vi "MultiPAS-IV_noCRD.vi"() -> ()   [LabVIEW 2011]
uses:
  <vilib>/Analysis/4window.llb/windowTd.ctl
  sub/QMH/QMH Add Message to Queue (Single Element).vi
  sub/QMH/QMH Add Message to Queue (Array).vi
  <vilib>/measure/maspectr.llb/FFT Spectrum (Mag-Phase) for 1 Chan.vi
  <vilib>/Instr/_visa.llb/VISA Configure Serial Port (Instr).vi
  <vilib>/measure/NI_MAPro.lvlib
  <vilib>/Analysis/NI_AALPro.lvlib
panel:
  in  "785 Power (mW)":dbl(slide)=100.0 min=0.0 max=100.0 step=1.0 scale=0.0..100.0
  in  "785 Emission":bool
  out "PAS Save":bool caption="Overtemp"
  in  "Data 2":i32[][](array[numeric])=[[-16374, -7248, 2543, 12030, 20279, 26487, 30037, 30583, 28073, 22744, 15131, 5976, -3818, -13288, -21504, -27663, -31155, -31636, -29064, -23686, -16036, -6862, 2936, 12388, 20571, 26684, 30122, 30546, 27911, 22483, 14793, 5595, -4207, -13644, -21795, -27855, -31232, -31591, -28898, -23423, -15695, -6476, 3323, 12743, 20858, 26873, 30194, 30492, 27744, 22213, 14447, 5207, -4597, -14002, -22082, -28044, -31304, -31540, -28731, -23149, -15348, -6093, 3713, 13101, 21145, 27063, 30265, 30442, 27576, 21943, 14103, 4822, -4984, -14354, -22365, -28230, -31373, -31485, -28556, -22876, -14998, -5702, 4104, 13452, 21428, 27245, 30335, 30388, 27400, 21669, 13754, 4435, -5375, -14705, -22643, -28407, -31436, -31426, -28378, -22598, -14648, -5314, 4497, 13803, 21706, 27423, 30394, 30325, 27221, 21390, 13402, 4045, -5763, -15056, -22921, -28586, -31496, -31361, -28198, -22319, -14297, -4924, 4879, 14151, 21982, 27597, 30451, 30257, 27038, 21107, 13050, 3658, -6149, -15402, -23193, -28754, -31546, -31290, -28010, -22033, -13944, -4536, 5266, 14498, 22252, 27767, 30500, 30184, 26849, 20821, 12696, 3267, -6535, -15748, -23462, -28924, -31596, -31216, -27821, -21748, -13587, -4147, 5653, 14838, 22519, 27930, 30549, 30110, 26658, 20535, 12337, 2878, -6919, -16089, -23727, -29087, -31641, -31137, -27627, -21457, -13229, -3753, 6038, 15181, 22786, 28093, 30591, 30031, 26461, 20243, 11979, 2485, -7303, -16428, -23991, -29244, -31678, -31053, -27426, -21159, -12867, -3360, 6424, 15524, 23043, 28252, 30633, 29946, 26262, 19946, 11617, 2096, -7686, -16764, -24246, -29398, -31712, -30964, -27224, -20862, -12503, -2971, 6803, 15859, 23301, 28401, 30661, 29852, 26058, 19648, 11254, 1703, -8069, -17099, -24500, -29547, -31741, -30870, -27018, -20562, -12138, -2575, 7188, 16192, 23556, 28549, 30689, 29756, 25848, 19348, 10891, 1312, -8448, -17430, -24753, -29691, -31765, -30773, -26806, -20259, -11775, -2186, 7566, 16521, 23801, 28690, 30709, 29656, 25634, 19038, 10523, 919, -8831, -17762, -24997, -29833, -31788, -30672, -26593, -19955, -11409, -1792, 7944, 16850, 24047, 28830, 30724, 29548, 25416, 18729, 10152, 523, -9212, -18092, -25245, -29969, -31805, -30566, -26375, -19647, -11041, -1403, 8319, 17173, 24287, 28963, 30734, 29436, 25192, 18418, 9781, 130, -9587, -18413, -25481, -30101, -31814, -30449, -26150, -19332, -10666, -1007, 8697, 17497, 24524, 29090, 30745, 29325, 24968, 18105, 9408, -263, -9962, -18735, -25718, -30228, -31820, -30334, -25921, -19016, -10296, -618, 9072, 17814, 24756, 29213, 30746, 29202, 24738, 17787, 9036, -657, -10338, -19058, -25951, -30350, -31818, -30214, -25690, -18699, -9922, -224, 9442, 18128, 24984, 29330, 30738, 29078, 24502, 17466, 8658, -1050, -10710, -19371, -26178, -30467, -31814, -30088, -25458, -18382, -9550, 167, 9812, 18440, 25206, 29443, 30732, 28947, 24264, 17143, 8281, -1445, -11083, -19685, -26404, -30581, -31807, -29959, -25221, -18059, -9175, 556, 10178, 18750, 25426, 29548, 30718, 28809, 24018, 16812, 7901, -1842, -11457, -19996, -26624, -30690, -31795, -29824, -24980, -17733, -8799, 950, 10549, 19058, 25643, 29655, 30700, 28673, 23773, 16484, 7523, -2235, -11824, -20304, -26840, -30793, -31772, -29682, -24731, -17402, -8415, 1341, 10916, 19363, 25856, 29755, 30677, 28528, 23522, 16151, 7141, -2626, -12191, -20607, -27051, -30891, -31746, -29536, -24481, -17070, -8035, 1733, 11280, 19664, 26064, 29851, 30648, 28381, 23272, 15818, 6762, -3019, -12555, -20906, -27258, -30984, -31717, -29391, -24226, -16736, -7655, 2128, 11641, 19962, 26270, 29940, 30615, 28229, 23013, 15483, 6376, -3409, -12914, -21204, -27459, -31071, -31684, -29236, -23967, -16398, -7271, 2515, 12005, 20258, 26468, 30024, 30577, 28072, 22753, 15143, 5990, -3802, -13276, -21497, -27660, -31157, -31643, -29076, -23707, -16058, -6886, 2908, 12363, 20550, 26666, 30107, 30536, 27914, 22489, 14805, 5607, -4192, -13633, -21787, -27849, -31230, -31597, -28911, -23438, -15716, -6501, 3298, 12719, 20839, 26858, 30182, 30488, 27744, 22223, 14459, 5225, -4579, -13988, -22071, -28040, -31304, -31549, -28743, -23167, -15368, -6113, 3693, 13076, 21126, 27047, 30255, 30438, 27576, 21950, 14113, 4837, -4971, -14340, -22354, -28224, -31375, -31494, -28570, -22895, -15022, -5725, 4080, 13430, 21408, 27230, 30324, 30384, 27402, 21676, 13766, 4449, -5360, -14694, -22636, -28409, -31440, -31436, -28397, -22617, -14674, -5338, 4467, 13781, 21686, 27408, 30385, 30320, 27224, 21398, 13418, 4062, -5748, -15044, -22913, -28584, -31498, -31368, -28212, -22339, -14321, -4948, 4856, 14131, 21963, 27583, 30440, 30254, 27042, 21118, 13062, 3669, -6137, -15390, -23183, -28751, -31551, -31297, -28024, -22049, -13962, -4556, 5245, 14476, 22235, 27754, 30497, 30186, 26857, 20834, 12710, 3283, -6519, -15733, -23453, -28921, -31600, -31226, -27837, -21765, -13610, -4168, 5628, 14820, 22502, 27918, 30540, 30109, 26664, 20544, 12354, 2891, -6906, -16074, -23719, -29085, -31646, -31148, -27642, -21475, -13251, -3777, 6014, 15160, 22765, 28078, 30583, 30027, 26468, 20251, 11994, 2501, -7292, -16415, -23980, -29242, -31682, -31064, -27443, -21181, -12892, -3386, 6397, 15501, 23026, 28238, 30624, 29944, 26269, 19959, 11633, 2110, -7673, -16753, -24239, -29395, -31719, -30974, -27239, -20882, -12528, -2993, 6782, 15835, 23285, 28390, 30651, 29852, 26063, 19660, 11271, 1720, -8053, -17087, -24493, -29546, -31746, -30880, -27031, -20583, -12163, -2599, 7166, 16173, 23538, 28538, 30684, 29758, 25853, 19356, 10906, 1327, -8433, -17416, -24743, -29688, -31769, -30782, -26821, -20280, -11797, -2208, 7543, 16501, 23786, 28680, 30704, 29656, 25642, 19053, 10540, 936, -8814, -17747, -24989, -29827, -31787, -30678, -26606, -19973, -11430, -1817, 7923, 16829, 24031, 28819, 30721, 29552, 25424, 18746, 10174, 543, -9191, -18072, -25231, -29962, -31802, -30567, -26384, -19660, -11057, -1422, 8302, 17159, 24274, 28952, 30738, 29443, 25205, 18435, 9801, 150, -9568, -18401, -25472, -30095, -31811, -30457, -26163, -19349, -10687, -1031, 8679, 17481, 24511, 29082, 30742, 29327, 24979, 18121, 9431, -241, -9943, -18717, -25707, -30221, -31815, -30337, -25930, -19029, -10312, -631, 9058, 17802, 24745, 29207, 30746, 29209, 24750, 17805, 9057, -634, -10316, -19037, -25937, -30340, -31814, -30217, -25700, -18713, -9939, -240, 9429, 18117, 24976, 29328, 30740, 29088, 24519, 17486, 8682, -1027, -10688, -19352, -26164, -30458, -31810, -30091, -25465, -18390, -9561, 154, 9800, 18433, 25201, 29442, 30735, 28959, 24282, 17165, 8308, -1420, -11063, -19665, -26386, -30570, -31801, -29961, -25227, -18068, -9185, 547, 10171, 18745, 25424, 29552, 30726, 28825, 24038, 16835, 7925, -1815, -11429, -19974, -26608, -30681, -31789, -29826, -24984, -17741, -8807, 938, 10536, 19047, 25636, 29657, 30708, 28685, 23794, 16510, 7550, -2205, -11798, -20280, -26821, -30782, -31766, -29684, -24737, -17411, -8429, 1331, 10906, 19356, 25851, 29758, 30684, 28544, 23546, 16178, 7169, -2598, -12162, -20582, -27035, -30879, -31744, -29540, -24485, -17080, -8048, 1721, 11267, 19655, 26061, 29852, 30654, 28395, 23291, 15843, 6786, -2993, -12527, -20884, -27240, -30974, -31713, -29390, -24230, -16744, -7662, 2115, 11635, 19957, 26268, 29945, 30624, 28246, 23035, 15509, 6406, -3382, -12889, -21180, -27444, -31061, -31677, -29236, -23975, -16408, -7284], [-19329, -1252, 17344, 29341, 30145, 19451, 1353, -17227, -29174, -29920, -19175, -1056, 17506, 29408, 30095, 19300, 1159, -17387, -29238, -29860, -19019, -860, 17671, 29475, 30037, 19143, 960, -17553, -29307, -29809, -18866, -664, 17832, 29545, 29987, 18991, 771, -17707, -29365, -29749, -18707, -466, 17992, 29605, 29926, 18832, 570, -17873, -29434, -29694, -18556, -272, 18151, 29670, 29869, 18676, 375, -18031, -29495, -29633, -18395, -75, 18310, 29729, 29809, 18516, 175, -18194, -29561, -29579, -18238, 120, 18469, 29792, 29750, 18362, -17, -18347, -29617, -29515, -18076, 316, 18629, 29848, 29682, 18197, -218, -18510, -29679, -29456, -17921, 513, 18787, 29910, 29626, 18042, -408, -18664, -29734, -29388, -17757, 709, 18941, 29965, 29560, 17875, -609, -18823, -29791, -29326, -17600, 904, 19095, 30023, 29495, 17717, -802, -18975, -29845, -29260, -17434, 1099, 19251, 30075, 29425, 17551, -1001, -19131, -29901, -29194, -17277, 1296, 19408, 30130, 29359, 17393, -1193, -19284, -29953, -29124, -17112, 1491, 19560, 30184, 29290, 17225, -1392, -19440, -30008, -29056, -16949, 1686, 19713, 30237, 29226, 17069, -1581, -19587, -30054, -28982, -16781, 1883, 19866, 30287, 29151, 16898, -1781, -19742, -30107, -28913, -16616, 2079, 20018, 30337, 29082, 16737, -1973, -19888, -30152, -28838, -16449, 2275, 20167, 30383, 29006, 16564, -2174, -20041, -30200, -28765, -16282, 2471, 20321, 30430, 28934, 16403, -2364, -20187, -30243, -28688, -16113, 2669, 20465, 30470, 28853, 16230, -2568, -20341, -30294, -28618, -15953, 2860, 20615, 30519, 28783, 16070, -2755, -20486, -30335, -28537, -15779, 3057, 20760, 30560, 28700, 15892, -2956, -20637, -30378, -28461, -15613, 3252, 20909, 30605, 28628, 15730, -3145, -20777, -30418, -28377, -15440, 3446, 21054, 30645, 28543, 15557, -3345, -20927, -30460, -28299, -15271, 3643, 21199, 30686, 28465, 15391, -3534, -21066, -30495, -28215, -15100, 3839, 21345, 30722, 28380, 15214, -3734, -21213, -30534, -28134, -14928, 4032, 21487, 30760, 28300, 15044, -3926, -21355, -30570, -28052, -14757, 4225, 21627, 30792, 28209, 14870, -4123, -21501, -30607, -27968, -14586, 4419, 21768, 30832, 28129, 14702, -4314, -21637, -30639, -27880, -14413, 4612, 21907, 30859, 28040, 14521, -4515, -21780, -30675, -27796, -14241, 4804, 22048, 30895, 27953, 14352, -4702, -21919, -30705, -27707, -14064, 4999, 22187, 30922, 27859, 14172, -4900, -22060, -30739, -27620, -13892, 5193, 22326, 30954, 27773, 14003, -5090, -22194, -30765, -27524, -13712, 5386, 22462, 30981, 27679, 13823, -5285, -22333, -30794, -27436, -13538, 5580, 22600, 31013, 27591, 13650, -5476, -22466, -30820, -27343, -13363, 5770, 22732, 31033, 27491, 13468, -5673, -22605, -30848, -27251, -13187, 5964, 22870, 31060, 27401, 13292, -5863, -22736, -30870, -27155, -13010, 6156, 23000, 31079, 27299, 13111, -6058, -22873, -30895, -27060, -12833, 6347, 23134, 31104, 27208, 12936, -6248, -23004, -30918, -26965, -12652, 6536, 23260, 31120, 27106, 12753, -6444, -23136, -30939, -26865, -12472, 6729, 23395, 31148, 27011, 12578, -6634, -23266, -30959, -26766, -12296, 6919, 23523, 31161, 26907, 12392, -6830, -23402, -30982, -26665, -12115, 7109, 23652, 31180, 26809, 12213, -7016, -23524, -30992, -26564, -11932, 7301, 23777, 31195, 26704, 12032, -7210, -23655, -31011, -26464, -11755, 7492, 23907, 31211, 26605, 11855, -7395, -23778, -31024, -26358, -11573, 7680, 24031, 31218, 26494, 11665, -7592, -23908, -31039, -26258, -11392, 7871, 24158, 31237, 26394, 11491, -7775, -24031, -31050, -26153, -11210, 8063, 24281, 31247, 26285, 11302, -7972, -24159, -31062, -26046, -11027, 8250, 24407, 31258, 26180, 11124, -8157, -24276, -31067, -25937, -10841, 8438, 24526, 31265, 26071, 10936, -8347, -24401, -31078, -25829, -10659, 8630, 24649, 31275, 25965, 10755, -8533, -24522, -31087, -25721, -10474, 8816, 24770, 31280, 25853, 10566, -8726, -24641, -31091, -25608, -10290, 9003, 24891, 31287, 25746, 10386, -8910, -24756, -31095, -25498, -10105, 9192, 25008, 31287, 25627, 10196, -9102, -24881, -31101, -25386, -9919, 9381, 25127, 31296, 25521, 10019, -9284, -24994, -31099, -25268, -9732, 9570, 25243, 31293, 25403, 9826, -9476, -25113, -31105, -25157, -9544, 9756, 25359, 31298, 25291, 9645, -9655, -25225, -31099, -25040, -9359, 9942, 25473, 31291, 25167, 9453, -9847, -25341, -31102, -24926, -9173, 10124, 25586, 31294, 25057, 9269, -10029, -25450, -31095, -24809, -8986, 10310, 25696, 31284, 24931, 9078, -10218, -25564, -31094, -24688, -8798, 10497, 25812, 31287, 24819, 8896, -10399, -25673, -31085, -24567, -8608, 10682, 25922, 31278, 24698, 8703, -10587, -25785, -31080, -24448, -8422, 10866, 26033, 31274, 24582, 8522, -10765, -25890, -31067, -24321, -8230, 11050, 26140, 31263, 24455, 8325, -10952, -26001, -31064, -24201, -8040, 11234, 26248, 31255, 24338, 8142, -11132, -26106, -31054, -24079, -7852, 11417, 26353, 31243, 24207, 7948, -11316, -26217, -31041, -23952, -7662, 11601, 26464, 31236, 24089, 7763, -11494, -26315, -31025, -23829, -7471, 11782, 26562, 31217, 23957, 7567, -11682, -26422, -31014, -23702, -7282, 11962, 26667, 31205, 23834, 7383, -11859, -26521, -30998, -23575, -7092, 12144, 26770, 31187, 23704, 7186, -12043, -26626, -30981, -23444, -6900, 12328, 26875, 31176, 23582, 7003, -12218, -26724, -30962, -23316, -6709, 12505, 26971, 31154, 23446, 6805, -12401, -26825, -30946, -23189, -6517, 12687, 27073, 31139, 23322, 6620, -12576, -26919, -30922, -23054, -6323, 12867, 27170, 31114, 23185, 6422, -12760, -27022, -30904, -22923, -6132, 13047, 27272, 31096, 23060, 6237, -12934, -27114, -30879, -22790, -5940, 13222, 27362, 31068, 22921, 6041, -13116, -27212, -30855, -22657, -5748, 13401, 27461, 31048, 22790, 5853, -13289, -27302, -30828, -22522, -5555, 13577, 27549, 31019, 22652, 5652, -13472, -27398, -30806, -22388, -5362, 13753, 27645, 30995, 22521, 5463, -13642, -27487, -30776, -22248, -5169, 13928, 27733, 30963, 22376, 5266, -13823, -27584, -30750, -22113, -4975, 14106, 27828, 30937, 22246, 5082, -13992, -27669, -30717, -21974, -4782, 14280, 27914, 30902, 22101, 4880, -14174, -27760, -30689, -21837, -4588, 14454, 28006, 30875, 21965, 4692, -14340, -27843, -30653, -21693, -4391, 14631, 28092, 30840, 21822, 4494, -14519, -27934, -30620, -21552, -4198, 14805, 28179, 30808, 21688, 4308, -14687, -28015, -30582, -21410, -4004, 14975, 28262, 30770, 21540, 4106, -14861, -28103, -30548, -21268, -3808, 15149, 28349, 30739, 21402, 3916, -15032, -28183, -30512, -21124, -3614, 15319, 28430, 30697, 21255, 3715, -15205, -28267, -30475, -20982, -3421, 15490, 28513, 30664, 21116, 3524, -15376, -28348, -30435, -20837, -3225, 15660, 28592, 30617, 20962, 3327, -15550, -28432, -30397, -20695, -3032, 15829, 28673, 30581, 20820, 3134, -15711, -28506, -30353, -20546, -2837, 15994, 28746, 30530, 20669, 2933, -15887, -28585, -30311, -20400, -2641, 16167, 28828, 30496, 20528, 2745, -16052, -28660, -30264, -20248, -2445, 16335, 28901, 30445, 20376, 2544, -16221, -28737, -30219, -20102, -2250, 16505, 28983, 30406, 20231, 2357, -16381, -28808, -30171, -19950, -2053, 16670, 29053, 30355, 20075, 2154, -16552, -28883, -30127, -19803, -1859, 16835, 29128, 30308, 19930, 1965, -16714, -28952, -30073, -19650, -1663, 17001, 29192, 30255, 19772, 1764, -16881, -29028, -30026, -19496, -1467, 17165, 29268, 30208, 19626, 1572, -17043, -29095, -29977, -19346]]
  out "Filtering":bool caption="Time has Elapsed"
  in  "Switch Filter":bool
  in  "Auto Filter":bool
  out "Elapsed Time (min)":dbl caption="Elapsed Time (s)" format="%#.1g"
  in  "Filter Length (min)":dbl=6.0 caption="Time Target (s)"
  in  "Sample Length (min)":dbl=24.0 caption="Time Target (s)" format="%#.1f"
  out "Time has Elapsed":bool
  in  "Time Target (s)":dbl=1.0
  out "PD Save":bool caption="Overtemp"
  in  "All Emit":bool
  in  "Alignment Mode":bool
  in  "660 Emission":bool
  in  "660 Power (mW)":dbl(slide)=100.0 min=0.0 max=100.0 step=1.0 scale=0.0..100.0
  in  "532 Emission":bool
  in  "532 Power (mW)":dbl(slide)=80.0 min=0.0 max=80.0 step=1.0 scale=0.0..80.0
  in  "405 Power (mW)":dbl(slide)=100.0 min=0.0 max=100.0 step=1.0 scale=0.0..100.0
  in  "405 Emission":bool
  out "Overtemp":bool
  in  "Tab Control":T1(tab)=enum."Frequency Sweep"
  in  "785 Port":refnum<visa-resource-name>="COM81"
  in  "Calibration Filepath":path
  in  "Save Cal?":bool=TRUE
  in  "pd id":u32=1
  in  "mic id":u32
  in  "mic cal, scu":dbl=5.41531278804282e-05 format="%#_3e"
  in  "mic cal, scu":dbl=5.59307241877627e-05 format="%#_3e"
  in  "405 Port":refnum<visa-resource-name>="COM80"
  in  "532 Port":refnum<visa-resource-name>="COM79"
  in  "660 Port":refnum<visa-resource-name>="COM62"
  in  "Teensy Port":refnum<visa-resource-name>="COM78"
  in  "Save Mic?":bool
  in  "Mic Time Series File Path":path
  out "error out":errorcluster
  in  "PD Time Series File Path":path
  in  "Save PD?":bool
  in  "Frequency Sweep File Path":path
  in  "Save sweeps?":bool
  in  "Save Abs?":bool
  in  "Abs Time Series File Path":path
  out "Laser Temperatures":T2
  in  "785 F (Hz)":i32=1370
  in  "check freqs?":bool=TRUE
  in  "autosweep":bool=TRUE
  in  "set freqs":bool
  out "Frequency Scan":cluster{i32[], "Best Gaussian Fit":dbl[]}[](graph)
  out "Calculated Resonance (Hz)":dbl=1370.0
  in  "Start (Hz)":i32=1355
  in  "End (Hz)":i32=1385
  out "Step No.":i32
  in  "405 F (Hz)":i32=1368
  in  "532 F (Hz)":i32=1372
  in  "660 F (Hz)":i32=1370
  in  "sweep laser?":bool=TRUE
  in  "sweep":bool
  in  "660 PD Cal 4":dbl=0.793
  in  "660 PD Cal 3":dbl=0.793
  in  "532 PD Cal 3":dbl=0.454
  in  "405 PD Cal 3":dbl=0.237
  out "PD Waveform":waveform(i32)(graph)
  out "PD FFT":cluster{"f0":dbl, "df":dbl, "magnitude":dbl[]}(graph)
  out "pd ts":cluster{dbl, dbl, dbl, dbl}(graph)
  in  "Chart Rolling Average Number\n(Transfers to Absorption Data!)":i32=1
  out "mic ts":T3(graph)
  out "Mic FFT":cluster{"f0":dbl, "df":dbl, "magnitude":dbl[]}(graph)
  out "Mic Waveform":waveform(i32)(graph)
  in  "calibrate":bool
  in  "GO3 Filepath":path=path "S:/Groups/Smith_G/Photoacoutic Spectroscopy/calibrations/20160810_cal_go3.txt"
  in  "Photodiode Filepath":path=path "S:/Groups/Smith_G/Photoacoutic Spectroscopy/calibrations/20160810_cal_pd.txt"
  in  "Microphone Filepath":path=path "S:/Groups/Smith_G/Photoacoutic Spectroscopy/calibrations/20160810_cal_mic.txt"
  in  "Bkg Start Index":i32=5
  out "aligned data":cluster{"Array":i32[], dbl[]}[](graph)
  out "Calibration":cluster{dbl[], dbl[]}[](graph)
  in  "Bkg End Index":i32=15
  in  "O3 Flow, sccm (80)":dbl=80.0
  in  "660 PD Cal":dbl=0.793
  in  "532 PD Cal":dbl=0.454
  out "532 Slope":dbl
  out "660 Slope":dbl
  out "PAS Cal Coefficient":dbl format="%0.2f"
  in  "GO3 Offset":i32=15
  in  "Cell Calibration, mV/mW":dbl=600000.0
  in  "getbkg":bool
  out "AAE":dbl(graph)
  in  "Bkg Values (mV)":cluster{dbl, dbl, dbl, dbl}
  out "Absorption Spectrum":cluster{dbl[], "Best Power Fit":dbl[]}[](graph)
  out "abs ts":cluster{dbl, dbl, dbl, dbl}(graph)
  out "Status":string
  in  "Exit":bool
  in  "State Variables":cluster{"CurrentFile":path}
  # "MultiPAS-IV | AeroSmith Labs (2016)"
  # "Laser Control"
  # "Filter Control"
  # "Communications"
  # "Sound Card Parameters"
  # "PD Calibration"
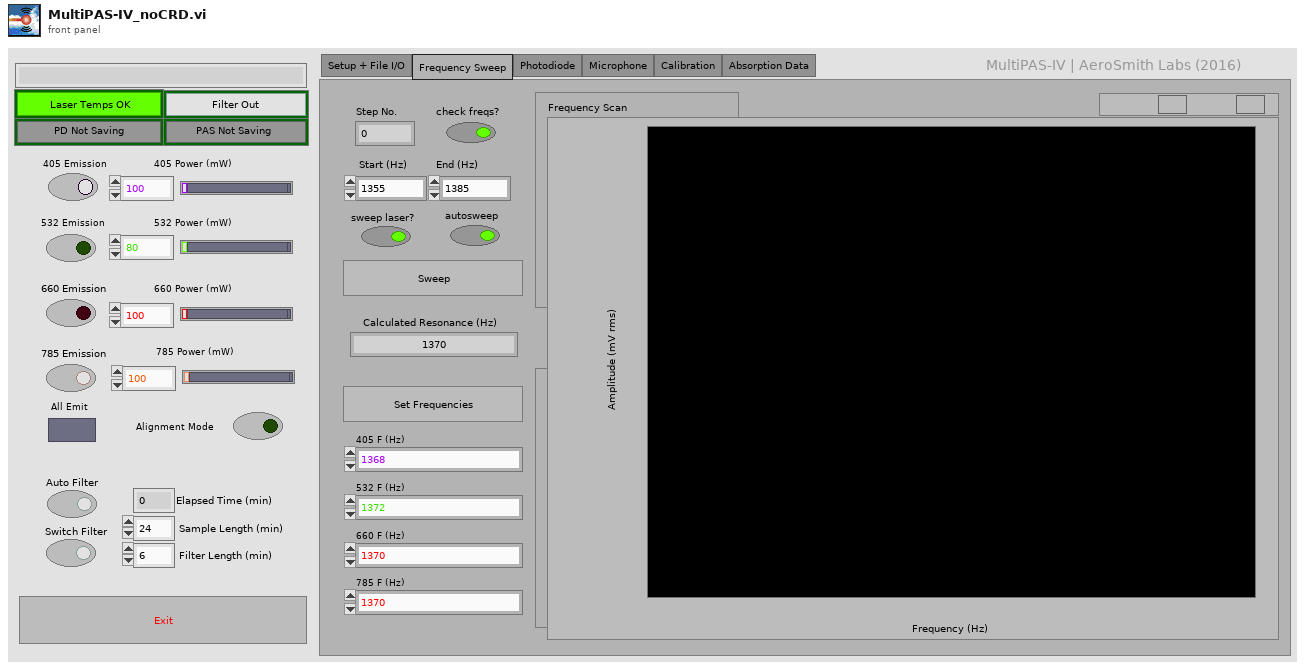
[diagram p1: front panel]
types:
  T1 = enum32{"Setup + File I/O", "Frequency Sweep", "Photodiode", "Microphone", "Calibration", "Absorption Data"}
  T2 = cluster{" 405 Temp (C)":dbl, "532 Temp (C)":dbl, "660 Temp (C)":dbl, "785 Temp (C)":dbl}
  T3 = cluster{"405 Mean":dbl, "532 Mean":dbl, "660 Mean":dbl, "785 Mean":dbl}
  T4 = cluster{"# buffers":i32, "Buffer size":i32, "unit (ms)":enum16{"time (ms)", "Samples"}}
  T5 = typedef "SoundHandle.ctl" = cluster{"DeviceID":u16, "Samples/buf":u32, "Sampl rate":u32, "Bits/sample":u16, "Channels":u8, "Opened":bool}
  T6 = typedef "NI_AALPro.lvlib/windowTd.ctl" = u32
  T7 = cluster{"785 New Array":dbl[], "785 Mean":dbl, "785 SD":dbl}
  T8 = cluster{"660 New Array":dbl[], "660 Mean":dbl, "660 SD":dbl}
  T9 = cluster{"532 New Array":dbl[], "532 Mean":dbl, "532 SD":dbl}
  T10 = cluster{"405 New Array":dbl[], "405 Mean":dbl, "405 SD":dbl}
  T11 = cluster{"Temp (C)":dbl, "Temp (C)":dbl, "Temp (C)":dbl, "Temp (C)":dbl}
  T12 = typedef "LVCursorListTypeDef.ctl" = cluster{"Name":string, "Color":u32, "Style":u8, "Point Style":u8, "Name Visible":bool, "Allow Drag":bool, "Cursor Mode":u32, "Plot":i32, "Index":i32, "Position":cluster{"X":dbl, "Y":dbl}, "X Scale":u32, "Y Scale":u32, "Watch Plots":i32[], "Watch All Plots":bool, "Plot Area":i32, "Label Offset":cluster{"X":dbl, "Y":dbl}}[]
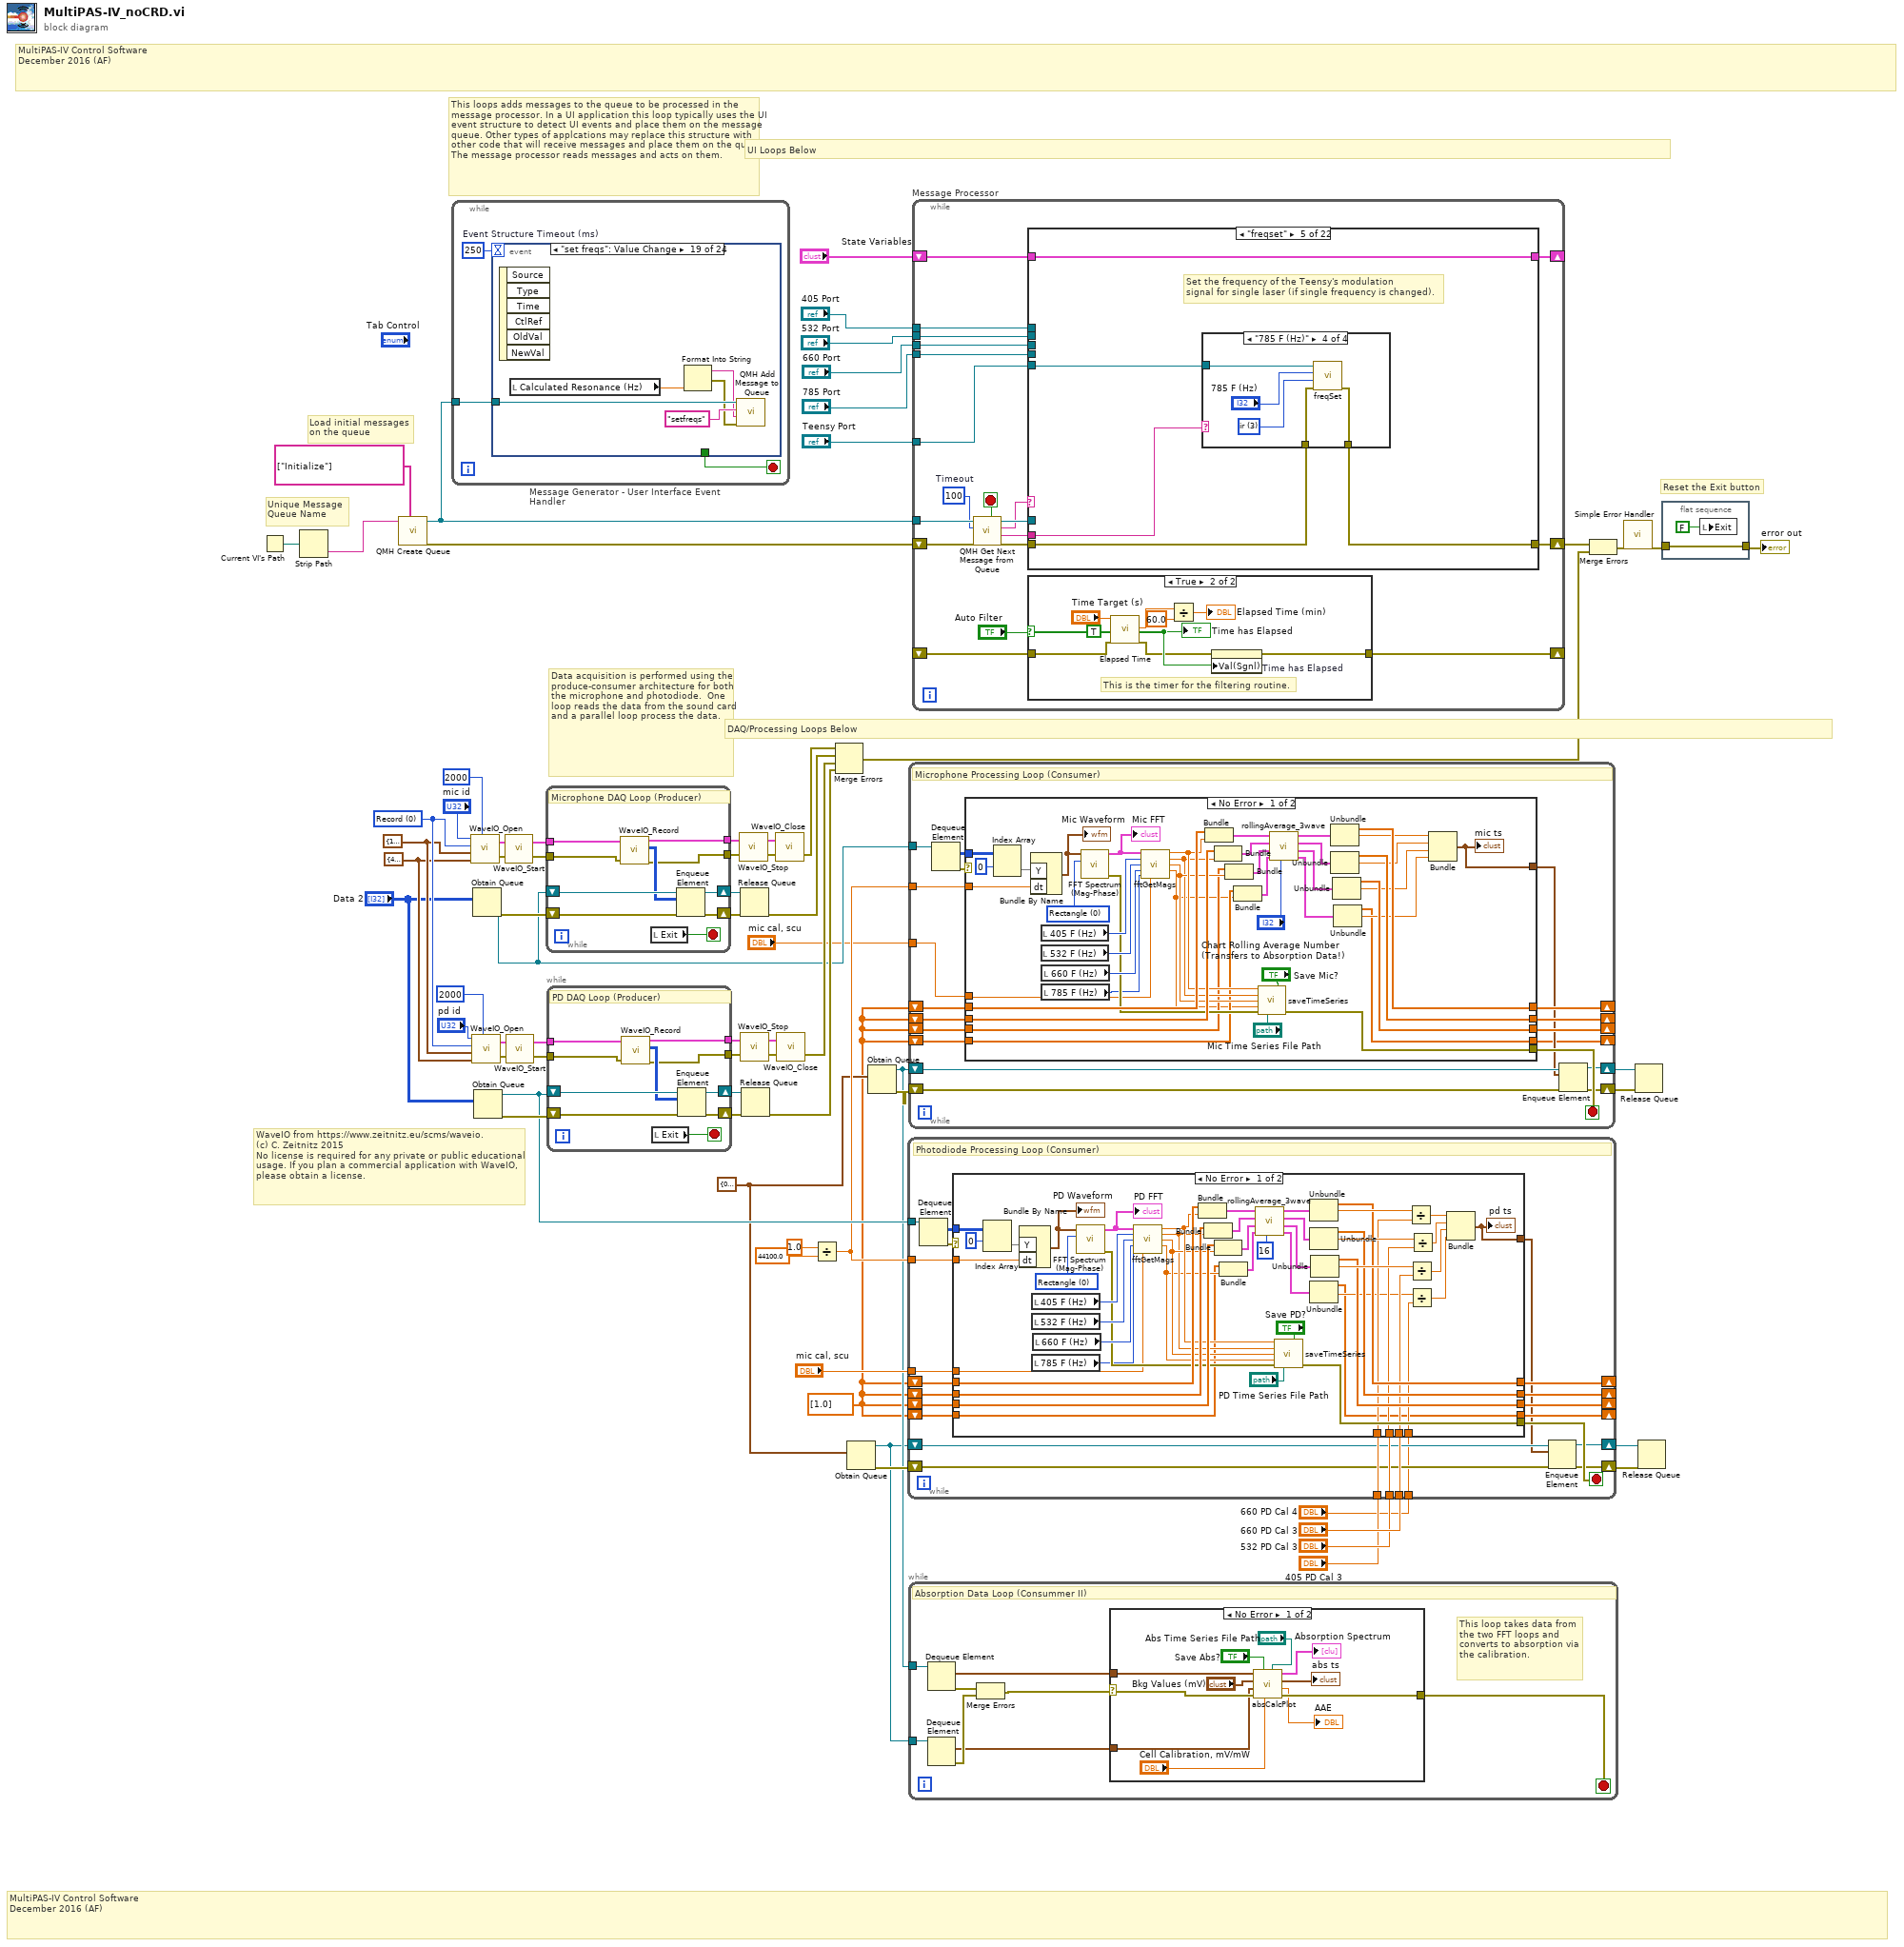
[diagram p0: block diagram]
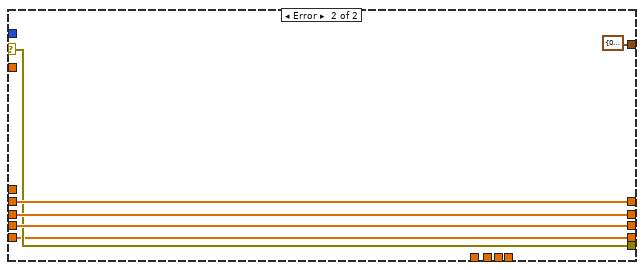
[diagram p3: hidden frame]
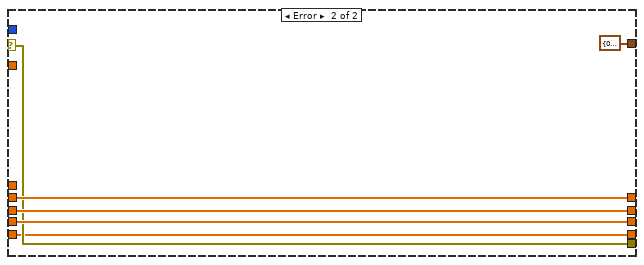
[diagram p4: hidden frame]
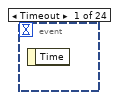
[diagram p5: hidden frame]
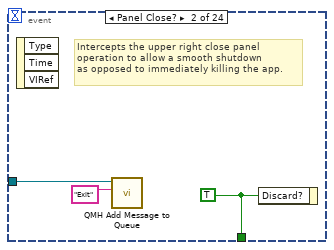
[diagram p6: hidden frame]
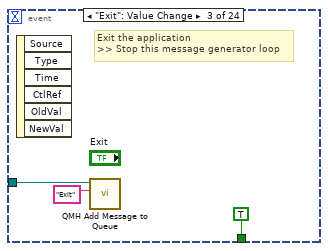
[diagram p7: hidden frame]
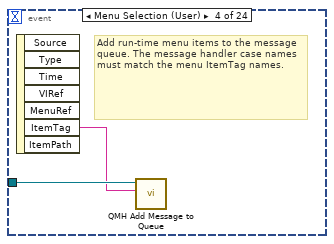
[diagram p8: hidden frame]
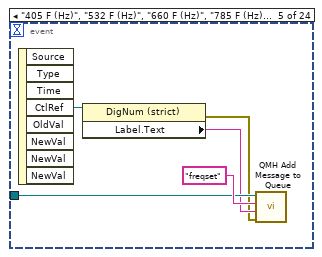
[diagram p9: hidden frame]
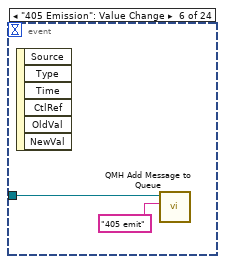
[diagram p10: hidden frame]
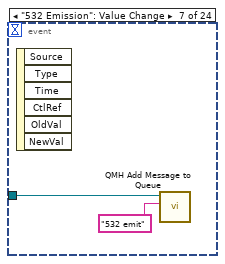
[diagram p11: hidden frame]
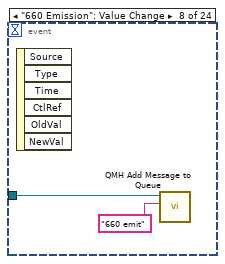
[diagram p12: hidden frame]
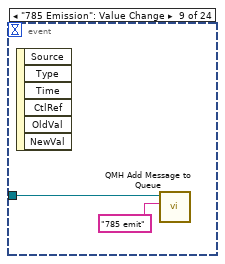
[diagram p13: hidden frame]
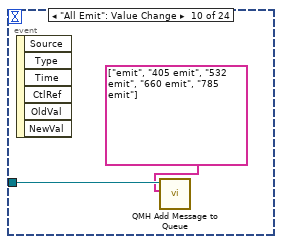
[diagram p14: hidden frame]
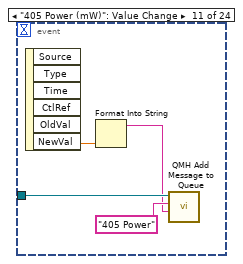
[diagram p15: hidden frame]
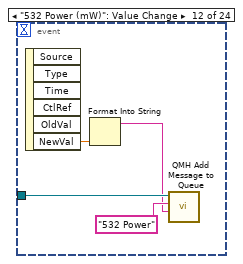
[diagram p16: hidden frame]
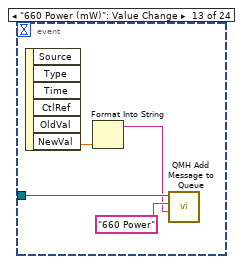
[diagram p17: hidden frame]
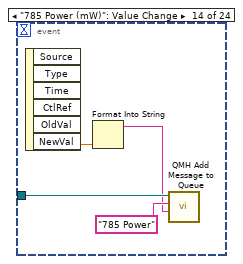
[diagram p18: hidden frame]
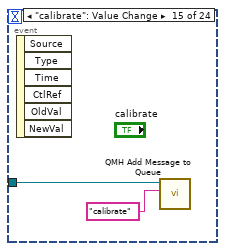
[diagram p19: hidden frame]
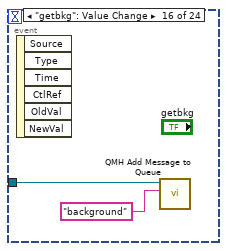
[diagram p20: hidden frame]
diagram:
  w3 = T3 {"405 Mean"=0.0, "532 Mean"=0.0, "660 Mean"=0.0, "785 Mean"=0.0} ("mic ts 2")
  w25 = T4 {"# buffers"=10, "Buffer size"=44100, "unit (ms)"=enum."Samples"} ("Buffer")
  w24 = cluster{"Rate":i32, "Bits":i32, "Channels":i32} {"Rate"=44100, "Bits"=24, "Channels"=2} ("Format")
  w26 = u16 0 items=["Record", "Play", "Loopback", "ASIO input", "ASIO output"] ("Direction (Record)")
  w2 = dbl[] [1.0] ("X")
  # "MultiPAS-IV Control Software\nDecember 2016 (AF)"
  # "MultiPAS-IV Control Software\nDecember 2016 (AF)"
  # "Data acquisition is performed using the produce-consumer architecture for both the microphone and photodiode.  One loop reads the data from the sound card and a parallel loop process the data."
  # "WaveIO from https://www.zeitnitz.eu/scms/waveio.\n(c) C. Zeitnitz 2015\nNo license is required for any private or public educational usage. If you plan a commercial application with WaveIO, please obtain a license."
  # "This loops adds messages to the queue to be processed in the message processor. In a UI application this loop typically uses the UI event structure to detect UI events and place them on the message queue. Other types of applcations may replace this structure with other code that will receive messages and place them on the queue.  The message processor reads messages and acts on them."
  # "Reset the Exit button"
  # "Unique Message\nQueue Name"
  # "Load initial messages\non the queue"
  # "DAQ/Processing Loops Below"
  # "UI Loops Below"
  n1 = Current VI's Path() -> (path=w70:path)
  n2 = Strip Path(path=w70) -> (name=w71:string)  [unwired: 1 out]
  n3 = call "QMH Create Queue.vi"("Initial Messages"=string[] ["Initialize"], "Message queue name (unnamed)"=w71) -> ("error out"=w67:errorcluster, "queue out"=w53:refnum<queue>)  [unwired: 8 in]
  n4 = while "Message Generator - User Interface Event Handler" {
    tunnel: w53 -> [w72]
    stop <- w73 stop-if-true
    w74 = 250  # Event Structure Timeout (ms)
    n5 = event shown="[18] \"set freqs\": Value Change" {
      selector: _ -> [_ _ _ _ _ _ _ _ _ _ _ _ _ _ _ _ _ _ _ _ _ _ _ _]
      dyn-events: _ -> [_ _ _ _ _ _ _ _ _ _ _ _ _ _ _ _ _ _ _ _ _ _ _ _]
      timeout: w74 -> [_ _ _ _ _ _ _ _ _ _ _ _ _ _ _ _ _ _ _ _ _ _ _ _]
      tunnel: [_ w77 TRUE ("Discard?") _ _ _ _ _ _ _ _ _ _ _ _ _ _ _ _ _ _ _ _ _] -> w73
      tunnel: w72 -> [_ w76 w79 w82 w86 w88 w90 w92 w94 w97 w100 w104 w108 w112 w114 w116 w118 w121 w125 _ _ w132 w136 w141]
      event Timeout {
        n6 = event-data() -> ()  [unwired: 1 in, 1 out]
      }
      event Panel Close? {
        w77 = TRUE ("Discard?")
        # "Intercepts the upper right close panel\noperation to allow a smooth shutdown\nas opposed to immediately killing the app."
        n7 = event-data() -> ()  [unwired: 1 in, 3 out]
        n8 = call-poly "QMH Add Message to Queue.vi"("Message"="Exit", "queue in"=w76) -> ()  [unwired: 8 in, 2 out]
        n9 = event-data("Discard?"=w77) -> ()  [unwired: 1 in, 1 out]
      }
      event "Exit": Value Change {
        # "Exit the application\n>> Stop this message generator loop"
        n10 = event-data() -> ()  [unwired: 1 in, 6 out]
        n11 = call-poly "QMH Add Message to Queue.vi"("Message"="Exit", "queue in"=w79) -> ()  [unwired: 8 in, 2 out]
      }
      event Menu Selection (User) {
        # "Add run-time menu items to the message\nqueue. The message handler case names must match the menu ItemTag names."
        n12 = event-data() -> ("ItemTag"=w81:string)  [unwired: 1 in, 6 out]
        n13 = call-poly "QMH Add Message to Queue.vi"("Message"=w81, "queue in"=w82) -> ()  [unwired: 8 in, 2 out]
      }
      event "405 F (Hz)", "532 F (Hz)", "660 F (Hz)", "785 F (Hz)": Value Change {
        n14 = event-data() -> ("CtlRef"=w85:refnum<vi>)  [unwired: 1 in, 7 out]
        n15 = property class="DigNum (strict)"(reference=w85) -> (error out=w83:errorcluster, "Label.Text"=w84:string)  [unwired: 1 in, 1 out]
        n16 = call-poly "QMH Add Message to Queue.vi"("error in (no error)"=w83, "Parameter"=w84, "Message"="freqset", "queue in"=w86) -> ()  [unwired: 6 in, 2 out]
      }
      event "405 Emission": Value Change {
        n17 = event-data() -> ()  [unwired: 1 in, 6 out]
        n18 = call-poly "QMH Add Message to Queue.vi"("Message"="405 emit", "queue in"=w88) -> ()  [unwired: 8 in, 2 out]
      }
      event "532 Emission": Value Change {
        n19 = event-data() -> ()  [unwired: 1 in, 6 out]
        n20 = call-poly "QMH Add Message to Queue.vi"("Message"="532 emit", "queue in"=w90) -> ()  [unwired: 8 in, 2 out]
      }
      event "660 Emission": Value Change {
        n21 = event-data() -> ()  [unwired: 1 in, 6 out]
        n22 = call-poly "QMH Add Message to Queue.vi"("Message"="660 emit", "queue in"=w92) -> ()  [unwired: 8 in, 2 out]
      }
      event "785 Emission": Value Change {
        n23 = event-data() -> ()  [unwired: 1 in, 6 out]
        n24 = call-poly "QMH Add Message to Queue.vi"("Message"="785 emit", "queue in"=w94) -> ()  [unwired: 8 in, 2 out]
      }
      event "All Emit": Value Change {
        n25 = event-data() -> ()  [unwired: 1 in, 6 out]
        n26 = call-poly "QMH Add Message to Queue.vi"("Messages"=string[] ["emit", "405 emit", "532 emit", "660 emit", "785 emit"], "queue in"=w97) -> ()  [unwired: 8 in, 2 out]
      }
      event "405 Power (mW)": Value Change {
        n27 = event-data() -> ("NewVal"=w99:dbl)  [unwired: 1 in, 5 out]
        n28 = Format Into String(w99) -> (resulting string=w98:string)  [unwired: 3 in, 1 out]
        n29 = call-poly "QMH Add Message to Queue.vi"("Parameter"=w98, "Message"="405 Power", "queue in"=w100) -> ()  [unwired: 7 in, 2 out]
      }
      event "532 Power (mW)": Value Change {
        n30 = event-data() -> ("NewVal"=w103:dbl)  [unwired: 1 in, 5 out]
        n31 = Format Into String(w103) -> (resulting string=w102:string)  [unwired: 3 in, 1 out]
        n32 = call-poly "QMH Add Message to Queue.vi"("Parameter"=w102, "Message"="532 Power", "queue in"=w104) -> ()  [unwired: 7 in, 2 out]
      }
      event "660 Power (mW)": Value Change {
        n33 = event-data() -> ("NewVal"=w107:dbl)  [unwired: 1 in, 5 out]
        n34 = Format Into String(w107) -> (resulting string=w106:string)  [unwired: 3 in, 1 out]
        n35 = call-poly "QMH Add Message to Queue.vi"("Parameter"=w106, "Message"="660 Power", "queue in"=w108) -> ()  [unwired: 7 in, 2 out]
      }
      event "785 Power (mW)": Value Change {
        n36 = event-data() -> ("NewVal"=w111:dbl)  [unwired: 1 in, 5 out]
        n37 = Format Into String(w111) -> (resulting string=w110:string)  [unwired: 3 in, 1 out]
        n38 = call-poly "QMH Add Message to Queue.vi"("Parameter"=w110, "Message"="785 Power", "queue in"=w112) -> ()  [unwired: 7 in, 2 out]
      }
      event "calibrate": Value Change {
        n39 = event-data() -> ()  [unwired: 1 in, 6 out]
        n40 = call-poly "QMH Add Message to Queue.vi"("Message"="calibrate", "queue in"=w114) -> ()  [unwired: 8 in, 2 out]
      }
      event "getbkg": Value Change {
        n41 = event-data() -> ()  [unwired: 1 in, 6 out]
        n42 = call-poly "QMH Add Message to Queue.vi"("Message"="background", "queue in"=w116) -> ()  [unwired: 8 in, 2 out]
      }
      event "Alignment Mode": Value Change {
        n43 = event-data() -> ()  [unwired: 1 in, 6 out]
        n44 = call-poly "QMH Add Message to Queue.vi"("Message"="align", "queue in"=w118) -> ()  [unwired: 8 in, 2 out]
      }
      event "sweep": Value Change {
        n45 = event-data() -> ()  [unwired: 1 in, 6 out]
        n46 = call-poly "QMH Add Message to Queue.vi"("Message"="sweep", "queue in"=w121) -> ()  [unwired: 8 in, 2 out]
      }
      event "set freqs": Value Change {
        n47 = event-data() -> ()  [unwired: 1 in, 6 out]
        n48 = local read "Calculated Resonance (Hz)"() -> (w124:dbl)
        n49 = Format Into String(w124) -> (resulting string=w123:string, error out=w122:errorcluster)  [unwired: 3 in]
        n50 = call-poly "QMH Add Message to Queue.vi"("error in (no error)"=w122, "Parameter"=w123, "Message"="setfreqs", "queue in"=w125) -> ()  [unwired: 6 in, 2 out]
      }
      event "Save Mic?": Value Change {
        n51 = event-data() -> ("NewVal"=→"PAS Save":bool)  [unwired: 1 in, 5 out]
      }
      event "Save PD?": Value Change {
        n52 = event-data() -> ("NewVal"=→"PD Save":bool)  [unwired: 1 in, 5 out]
      }
      event "Switch Filter": Value Change {
        n53 = event-data() -> ("NewVal"=w131:bool)  [unwired: 1 in, 5 out]
        n54 = local write "Filtering"(w131) -> ()
        n55 = Format Into String(w131) -> (resulting string=w129:string)  [unwired: 3 in, 1 out]
        n56 = call-poly "QMH Add Message to Queue.vi"("Parameter"=w129, "Message"="filterswitch", "queue in"=w132) -> ()  [unwired: 7 in, 2 out]
      }
      event "Time has Elapsed": Value Change {
        n57 = event-data() -> ("NewVal"=w135:bool)  [unwired: 1 in, 5 out]
        n58 = local read "Filtering"() -> (w134:bool)
        n59 = call "filterCreateMsg.vi"("time elapsed?"=w135, "auto sweep (true)"="autosweep", "filtering (true)"=w134, "queue in"=w136) -> ()  [unwired: 6 in, 2 out]
      }
      event "Calculated Resonance (Hz)": Value Change {
        n60 = event-data() -> ("NewVal"=w139:dbl)  [unwired: 1 in, 5 out]
        n61 = Format Into String(w139) -> (resulting string=w137:string, error out=w138:errorcluster)  [unwired: 3 in]
        n62 = call-poly "QMH Add Message to Queue.vi"("error in (no error)"=w138, "Parameter"=w137, "Message"="setfreqs", "queue in"=w141) -> ()  [unwired: 6 in, 2 out]
      }
    }
  }
  n63 = call <userlib>:"WaveIO_Open.vi"("Watchdog timeout (msec) (default=OFF)"=2000, "Format (44kHz, 16Bit, stereo)"=w24, "Buffer Config"=w25, "Direction (Record)"=w26, "idev"="mic id") -> ("error out"=w49:errorcluster, "Sound Handle Out"=w50:T5)  [unwired: 1 in]
  n64 = call <userlib>:"WaveIO_Open.vi"("Watchdog timeout (msec) (default=OFF)"=2000, "Format (44kHz, 16Bit, stereo)"=w24, "Buffer Config"=w25, "Direction (Record)"=w26, "idev"="pd id") -> ("error out"=w35:errorcluster, "Sound Handle Out"=w34:T5)  [unwired: 1 in]
  n65 = Obtain Queue(element data type="Data 2") -> (queue out=w18:refnum<queue>, error out=w56:errorcluster)  [unwired: 4 in, 1 out]
  n66 = Obtain Queue(element data type="Data 2") -> (queue out=w22:refnum<queue>, error out=w31:errorcluster)  [unwired: 4 in, 1 out]
  n67 = call <userlib>:"WaveIO_Start.vi"("error in (no error)"=w49, "Handle"=w50) -> ("error out"=w47:errorcluster, "Handle Out"=w48:T5)
  n68 = call <userlib>:"WaveIO_Start.vi"("error in (no error)"=w35, "Handle"=w34) -> ("error out"=w37:errorcluster, "Handle Out"=w36:T5)
  n69 = while {
    shift-right: [w150] -> w57
    shift-left: w18 -> [w148]
    shift-right: [w151] -> w58
    shift-left: w56 -> [w149]
    tunnel: w48 -> [w146]
    tunnel: w47 -> [w145]
    tunnel: [w143] -> w44
    tunnel: [w142] -> w43
    stop <- w147 stop-if-true
    # "Microphone DAQ Loop (Producer)"
    n70 = call <userlib>:"WaveIO_Record.vi"("Handle"=w146, "error in (no error)"=w145) -> ("Handle Out"=w143:T5, "Data"=w144:i32[][], "error out"=w142:errorcluster)  [unwired: 1 in, 2 out]
    n71 = local read "Exit"() -> (w147:bool)
    n72 = Enqueue Element(queue=w148, element=w144, error in (no error)=w149) -> (queue out=w150:refnum<queue>, error out=w151:errorcluster)  [unwired: 1 in, 1 out]
  }
  n73 = while {
    shift-right: [w160] -> w30
    shift-left: w22 -> [w158]
    shift-right: [w161] -> w29
    shift-left: w31 -> [w159]
    tunnel: w36 -> [w156]
    tunnel: w37 -> [w155]
    tunnel: [w153] -> w40
    tunnel: [w152] -> w41
    stop <- w157 stop-if-true
    # "PD DAQ Loop (Producer)"
    n74 = call <userlib>:"WaveIO_Record.vi"("Handle"=w156, "error in (no error)"=w155) -> ("Handle Out"=w153:T5, "Data"=w154:i32[][], "error out"=w152:errorcluster)  [unwired: 1 in, 2 out]
    n75 = local read "Exit"() -> (w157:bool)
    n76 = Enqueue Element(queue=w158, element=w154, error in (no error)=w159) -> (queue out=w160:refnum<queue>, error out=w161:errorcluster)  [unwired: 1 in, 1 out]
  }
  n77 = call <userlib>:"WaveIO_Stop.vi"("error in (no error)"=w43, "Handle"=w44) -> ("error out"=w45:errorcluster, "Handle Out"=w46:T5)
  n78 = Release Queue(queue=w57, error in (no error)=w58) -> (error out=w55:errorcluster)  [unwired: 1 in, 2 out]
  n79 = call <userlib>:"WaveIO_Stop.vi"("error in (no error)"=w41, "Handle"=w40) -> ("error out"=w39:errorcluster, "Handle Out"=w38:T5)
  n80 = Release Queue(queue=w30, error in (no error)=w29) -> (error out=w28:errorcluster)  [unwired: 1 in, 2 out]
  n81 = call <userlib>:"WaveIO_Close.vi"("error in (no error)"=w45, "Handle"=w46) -> ("error out"=w42:errorcluster)  [unwired: 1 out]
  n82 = call <userlib>:"WaveIO_Close.vi"("error in (no error)"=w39, "Handle"=w38) -> ("error out"=w27:errorcluster)  [unwired: 1 out]
  n83 = Divide(x=1.0, y=44100.0) -> (x/y=w19:dbl)
  n84 = Merge Errors(w42, w55, w27, w28) -> (w54:errorcluster)
  n85 = Obtain Queue(element data type=w3) -> (queue out=w5:refnum<queue>, error out=w9:errorcluster)  [unwired: 4 in, 1 out]
  n86 = Obtain Queue(element data type=w3) -> (queue out=w6:refnum<queue>, error out=w12:errorcluster)  [unwired: 4 in, 1 out]
  n87 = while {
    shift-right: [w182] -> _
    shift-left: w2 -> [w179]
    shift-right: [w181] -> _
    shift-left: w2 -> [w178]
    shift-right: [w180] -> _
    shift-left: w2 -> [w177]
    tunnel: w22 -> [w175]
    tunnel: w19 -> [w174]
    tunnel: "mic cal, scu" -> [w173]
    tunnel: "660 PD Cal 3" -> [w172]
    tunnel: "532 PD Cal 3" -> [w171]
    tunnel: "405 PD Cal 3" -> [w170]
    shift-right: [w167] -> w8
    shift-left: w5 -> [w168]
    shift-right: [w166] -> w7
    shift-left: w9 -> [w169]
    shift-right: [w163] -> _
    shift-left: w2 -> [w165]
    tunnel: "660 PD Cal 4" -> [w164]
    stop <- w176 stop-if-true
    # "Photodiode Processing Loop (Consumer)"
    n88 = Dequeue Element(queue=w175) -> (element=w183:i32[][], error out=w184:errorcluster)  [unwired: 2 in, 2 out]
    n89 = case shown="No Error" w184 {
      selector: w184 -> [_ w237]
      tunnel: w183 -> [w204 _]
      tunnel: w179 -> [w229 w240]
      tunnel: w178 -> [w228 w238]
      tunnel: w177 -> [w227 w239]
      tunnel: [w211 w240] -> w182
      tunnel: [w210 w238] -> w181
      tunnel: [w209 w239] -> w180
      tunnel: [w208 w237] -> w176
      tunnel: w174 -> [w201 _]
      tunnel: w173 -> [w199 _]
      tunnel: w172 -> [w198 _]
      tunnel: w171 -> [w197 _]
      tunnel: w170 -> [w196 _]
      tunnel: [w195 T3 {"405 Mean"=0.0, "532 Mean"=0.0, "660 Mean"=0.0, "785 Mean"=0.0} ("mic ts 2")] -> w162
      tunnel: w165 -> [w193 w236]
      tunnel: w164 -> [w189 _]
      tunnel: [w187 w236] -> w163
      frame No Error {
        w231 = T6 0 items=["Rectangle"=0, "Hanning"=1, "Hamming"=2, "Blackman-Harris"=3, "Exact Blackman"=4, "Blackman"=5, "Flat Top"=6, "4 Term B-Harris "=7, "7 Term B-Harris"=8, "Low Sidelobe"=9, "Blackman Nuttall"=11, "Triangle"=30, "Bartlett-Hanning"=31, "Bohman"=32, "Parzen"=33, "Welch"=34, "Kaiser"=60, "Dolph-Chebyshev"=61, "Gaussian"=62] ("window")
        n90 = Index Array(array=w204, index (row)=0) -> (element=w203:i32[])  [unwired: 1 in]
        n91 = Bundle By Name("Y"=w203, "dt"=w201) -> (w202:waveform(i32))  [unwired: 1 in]
        "PD Waveform" <- w202
        n92 = local read "405 F (Hz)"() -> (w234:i32)
        n93 = local read "532 F (Hz)"() -> (w233:i32)
        n94 = local read "785 F (Hz)"() -> (w185:i32)
        n95 = local read "660 F (Hz)"() -> (w232:i32)
        n96 = call-poly <vilib>:"FFT Spectrum (Mag-Phase).vi"("window"=w231, "time signal"=w202) -> ("error out"=w223:errorcluster, "magnitude"=w200:cluster{"f0":dbl, "df":dbl, "magnitude":dbl[]})  [unwired: 5 in, 3 out]
        "PD FFT" <- w200
        n97 = call "fftGetMags.vi"("input cluster"=w200, "405 F (Hz)"=w234, "532 F (Hz)"=w233, "660 F (Hz)"=w232, "785 F (Hz)"=w185, "unit cal, scu"=w199) -> ("mag405 (mV)"=w226:dbl, "mag532 (mV)"=w224:dbl, "mag660 (mV)"=w225:dbl, "mag785 (mV)"=w194:dbl)  [unwired: 6 in]
        n98 = Bundle("X"=w229, "mag405 (mV)"=w226) -> (w230:cluster{"X":dbl[], "mag405 (mV) ":dbl})  [unwired: 1 in]
        n99 = Bundle("X"=w228, "mag532 (mV)"=w224) -> (w222:cluster{"X":dbl[], "mag532 (mV)":dbl})  [unwired: 1 in]
        n100 = Bundle("X"=w227, "mag660 (mV)"=w225) -> (w221:cluster{"X":dbl[], "mag660 (mV)":dbl})  [unwired: 1 in]
        n101 = Bundle("X"=w193, "mag785 (mV)"=w194) -> (w192:cluster{"X":dbl[], "mag785 (mV)":dbl})  [unwired: 1 in]
        n102 = call "rollingAverage_3wave.vi"("Magnitude Averaging (no. Avgs.)"=16, "785"=w192, "660"=w221, "532"=w222, "405"=w230) -> ("785 Data"=w190:T7, "660 Data"=w212:T8, "532 Data"=w213:T9, "405 Data"=w214:T10)  [unwired: 3 in]
        n103 = call "saveTimeSeries.vi"("405nm"=w226, "file path (dialog if empty)"="PD Time Series File Path", "save?"="Save PD?", "532nm"=w224, "660nm"=w225, "785nm"=w194, "Error In"=w223) -> ("Error Out"=w208:errorcluster)  [unwired: 8 in]
        n104 = Unbundle(w214) -> ("405 New Array"=w211:dbl[], "405 Mean"=w219:dbl)  [unwired: 1 out]
        n105 = Unbundle(w213) -> ("532 New Array"=w210:dbl[], "532 Mean"=w217:dbl)  [unwired: 1 out]
        n106 = Unbundle(w190) -> ("785 New Array"=w187:dbl[], "785 Mean"=w188:dbl)  [unwired: 1 out]
        n107 = Unbundle(w212) -> ("660 New Array"=w209:dbl[], "660 Mean"=w215:dbl)  [unwired: 1 out]
        n108 = Divide(x=w219, y=w196) -> (x/y=w220:dbl)
        n109 = Divide(x=w215, y=w198) -> (x/y=w216:dbl)
        n110 = Divide(x=w188, y=w189) -> (x/y=w186:dbl)
        n111 = Divide(x=w217, y=w197) -> (x/y=w218:dbl)
        n112 = Bundle(w220, w218, w216, w186) -> (w195:cluster{dbl, dbl, dbl, dbl})  [unwired: 1 in]
        "pd ts" <- w195
      }
      frame Error {
      }
    }
    n113 = Enqueue Element(queue=w168, element=w162, error in (no error)=w169) -> (queue out=w167:refnum<queue>, error out=w166:errorcluster)  [unwired: 1 in, 1 out]
  }
  n114 = while {
    tunnel: w18 -> [w259]
    shift-right: [w256] -> _
    shift-left: w2 -> [w253]
    shift-right: [w255] -> _
    shift-left: w2 -> [w252]
    shift-right: [w254] -> _
    shift-left: w2 -> [w251]
    tunnel: w19 -> [w249]
    tunnel: "mic cal, scu" -> [w248]
    shift-right: [w246] -> w11
    shift-left: w6 -> [w245]
    shift-right: [w243] -> w10
    shift-left: w12 -> [w247]
    shift-right: [w241] -> _
    shift-left: w2 -> [w242]
    stop <- w250 stop-if-true
    # "Microphone Processing Loop (Consumer)"
    n115 = Dequeue Element(queue=w259) -> (element=w257:i32[][], error out=w258:errorcluster)  [unwired: 2 in, 2 out]
    n116 = case shown="No Error" w258 {
      selector: w258 -> [_ w304]
      tunnel: w257 -> [w278 _]
      tunnel: w253 -> [w296 w307]
      tunnel: w252 -> [w295 w305]
      tunnel: w251 -> [w266 w306]
      tunnel: [w285 w307] -> w256
      tunnel: [w284 w305] -> w255
      tunnel: [w283 w306] -> w254
      tunnel: [w282 w304] -> w250
      tunnel: w249 -> [w275 _]
      tunnel: w248 -> [w273 _]
      tunnel: [w269 T3 {"405 Mean"=0.0, "532 Mean"=0.0, "660 Mean"=0.0, "785 Mean"=0.0} ("mic ts 2")] -> w244
      tunnel: w242 -> [w267 w302]
      tunnel: [w260 w302] -> w241
      frame No Error {
        w298 = T6 0 items=["Rectangle"=0, "Hanning"=1, "Hamming"=2, "Blackman-Harris"=3, "Exact Blackman"=4, "Blackman"=5, "Flat Top"=6, "4 Term B-Harris "=7, "7 Term B-Harris"=8, "Low Sidelobe"=9, "Blackman Nuttall"=11, "Triangle"=30, "Bartlett-Hanning"=31, "Bohman"=32, "Parzen"=33, "Welch"=34, "Kaiser"=60, "Dolph-Chebyshev"=61, "Gaussian"=62] ("window")
        n117 = Index Array(array=w278, index (row)=0) -> (element=w277:i32[])  [unwired: 1 in]
        n118 = Bundle By Name("Y"=w277, "dt"=w275) -> (w276:waveform(i32))  [unwired: 1 in]
        "Mic Waveform" <- w276
        n119 = local read "405 F (Hz)"() -> (w301:i32)
        n120 = local read "532 F (Hz)"() -> (w300:i32)
        n121 = local read "660 F (Hz)"() -> (w299:i32)
        n122 = local read "785 F (Hz)"() -> (w268:i32)
        n123 = call-poly <vilib>:"FFT Spectrum (Mag-Phase).vi"("window"=w298, "time signal"=w276) -> ("error out"=w291:errorcluster, "magnitude"=w274:cluster{"f0":dbl, "df":dbl, "magnitude":dbl[]})  [unwired: 5 in, 3 out]
        "Mic FFT" <- w274
        n124 = call "fftGetMags.vi"("input cluster"=w274, "405 F (Hz)"=w301, "532 F (Hz)"=w300, "660 F (Hz)"=w299, "785 F (Hz)"=w268, "unit cal, scu"=w273) -> ("mag405 (mV)"=w294:dbl, "mag532 (mV)"=w292:dbl, "mag660 (mV)"=w293:dbl, "mag785 (mV)"=w265:dbl)  [unwired: 6 in]
        n125 = Bundle("X"=w296, "mag405 (mV)"=w294) -> (w297:cluster{"X":dbl[], "mag405 (mV) ":dbl})  [unwired: 1 in]
        n126 = Bundle("X"=w295, "mag532 (mV)"=w292) -> (w290:cluster{"X":dbl[], "mag532 (mV)":dbl})  [unwired: 1 in]
        n127 = Bundle("X"=w266, "mag660 (mV)"=w293) -> (w289:cluster{"X":dbl[], "mag660 (mV)":dbl})  [unwired: 1 in]
        n128 = Bundle("X"=w267, "mag785 (mV)"=w265) -> (w263:cluster{"X":dbl[], "mag785 (mV)":dbl})  [unwired: 1 in]
        n129 = call "saveTimeSeries.vi"("405nm"=w294, "file path (dialog if empty)"="Mic Time Series File Path", "save?"="Save Mic?", "532nm"=w292, "660nm"=w293, "785nm"=w265, "Error In"=w291) -> ("Error Out"=w282:errorcluster)  [unwired: 8 in]
        n130 = call "rollingAverage_3wave.vi"("Magnitude Averaging (no. Avgs.)"="Chart Rolling Average Number\n(Transfers to Absorption Data!)", "785"=w263, "660"=w289, "532"=w290, "405"=w297) -> ("785 Data"=w262:T7, "660 Data"=w286:T8, "532 Data"=w287:T9, "405 Data"=w288:T10)  [unwired: 3 in]
        n131 = Unbundle(w288) -> ("405 New Array"=w285:dbl[], "405 Mean"=w272:dbl)  [unwired: 1 out]
        n132 = Unbundle(w287) -> ("532 New Array"=w284:dbl[], "532 Mean"=w271:dbl)  [unwired: 1 out]
        n133 = Unbundle(w286) -> ("660 New Array"=w283:dbl[], "660 Mean"=w270:dbl)  [unwired: 1 out]
        n134 = Unbundle(w262) -> ("785 New Array"=w260:dbl[], "785 Mean"=w261:dbl)  [unwired: 1 out]
        n135 = Bundle("405 Mean"=w272, "532 Mean"=w271, "660 Mean"=w270, "785 Mean"=w261) -> (w269:T3)  [unwired: 1 in]
        "mic ts" <- w269
      }
      frame Error {
      }
    }
    n136 = Enqueue Element(queue=w245, element=w244, error in (no error)=w247) -> (queue out=w246:refnum<queue>, error out=w243:errorcluster)  [unwired: 1 in, 1 out]
  }
  n137 = while {
    tunnel: w6 -> [w309]
    tunnel: w5 -> [w308]
    stop <- w314 stop-if-true
    # "This loop takes data from the two FFT loops and converts to absorption via the calibration."
    # "Absorption Data Loop (Consummer II)"
    n138 = Dequeue Element(queue=w309) -> (element=w315:T3, error out=w313:errorcluster)  [unwired: 2 in, 2 out]
    n139 = Dequeue Element(queue=w308) -> (element=w310:T3, error out=w312:errorcluster)  [unwired: 2 in, 2 out]
    n140 = Merge Errors(w313, w312) -> (w311:errorcluster)
    n141 = case shown="No Error" w311 {
      selector: w311 -> [w322 w327]
      tunnel: w315 -> [w317 _]
      tunnel: [w321 w327] -> w314
      tunnel: w310 -> [w316 _]
      frame No Error {
        n142 = call "absCalcPlot.vi"("file path (dialog if empty)"="Abs Time Series File Path", "Cell Calibration, mV/mW"="Cell Calibration, mV/mW", "save?"="Save Abs?", "Error In"=w322, "PD Values"=w316, "bkg values"="Bkg Values (mV)", "Mic Values"=w317) -> ("Error Out"=w321:errorcluster, "aae"=→"AAE":dbl, "Time Series"=→"abs ts":cluster{dbl, dbl, dbl, dbl}, "Spectrum"=→"Absorption Spectrum":cluster{dbl[], "Best Power Fit":dbl[]}[])  [unwired: 1 in]
      }
      frame Error {
      }
    }
  }
  n143 = while "Message Processor" {
    shift-left: w67 -> [w341]
    shift-right: [w333] -> w63
    tunnel: w53 -> [w340]
    shift-left: "State Variables" -> [w346]
    shift-right: [w345] -> _
    tunnel: "405 Port" -> [w337]
    tunnel: "532 Port" -> [w336]
    tunnel: "660 Port" -> [w335]
    tunnel: "Teensy Port" -> [w334]
    shift-right: [w331] -> _
    shift-left: _ -> [w330]
    tunnel: "785 Port" -> [w328]
    stop <- w344 stop-if-true
    w338 = 100  # Timeout
    n144 = call "QMH Get Next Message from Queue.vi"("error in (no error)"=w341, "ms timeout (1)"=w338, "queue in"=w340) -> ("error out"=w342:errorcluster, "Next Parameter"=w329:string, "Next Message"=w339:string, "queue out"=w343:refnum<queue>, "Stop QMH"=w344:bool)  [unwired: 3 in]
    n145 = case shown="\"freqset\"" w339 {
      selector: w339 -> [_ w374 _ _ _ _ _ _ _ _ _ _ _ _ _ _ _ _ _ _ _ _]
      tunnel: [w370 w375 w388 w399 w459 w487 w529 w536 w542 w550 w554 w560 w568 w575 w582 w590 w615 w622 w646 w665 w694 w706] -> w345
      tunnel: w346 -> [w370 w375 w388 w399 w459 w487 w529 w536 w542 w550 w554 w560 w568 w575 w582 w590 w615 w622 w646 w665 w694 w706]
      tunnel: w343 -> [_ _ _ w392 _ _ _ _ _ _ _ _ _ _ _ _ _ _ _ _ w692 w707]
      tunnel: w342 -> [w361 w371 w386 w398 w457 w482 w532 w538 w544 w551 w553 w556 w565 w572 w579 w588 w616 w619 w644 w666 w693 w708]
      tunnel: [w359 w371 w380 w391 w456 w484 w528 w534 w540 w549 w553 w559 w566 w573 w580 w584 w616 w618 w643 w666 w690 w697] -> w333
      tunnel: w337 -> [w364 _ w387 w390 _ _ w531 _ _ _ _ w561 _ _ _ w587 _ _ _ _ _ w703]
      tunnel: w336 -> [w363 _ w384 w394 _ _ _ w535 _ _ _ _ w567 _ _ w586 _ _ _ _ _ w702]
      tunnel: w335 -> [w358 _ w383 w397 _ _ _ _ w541 _ _ _ _ w574 w581 w585 _ _ _ _ _ w701]
      tunnel: w334 -> [_ _ w381 w393 w458 w485 _ _ _ _ _ _ _ _ _ _ _ w620 w645 _ _ w704]
      tunnel: w329 -> [_ _ _ _ w455 w480 _ _ _ _ _ w558 w562 w569 w576 _ _ _ w642 _ _ _]
      tunnel: w328 -> [w357 _ w379 w389 _ _ _ _ _ w546 _ _ _ _ _ w583 _ _ _ _ _ w695]
      frame "", "Wait" {
        # "Update the front panel"
        # "Idle Case - this case is called after a Timeout on the Get Next Message from Queue VI, if no new messages are present on the queue. This case can be used for housekeeping tasks such as updating the UI."
        n146 = Get Date/Time String(want seconds? (F)=TRUE) -> (date string=w369:string, time string=w368:string)  [unwired: 2 in]
        n147 = call "laserDiagnose.vi"("405 Port"=w364, "532 Port"=w363, "660 Port"=w358, "785 Port"=w357, "error in (no error)"=w361) -> ("Temperatures"=→"Laser Temperatures":T11, "Overtemp"=→"Overtemp":bool, "error out"=w359:errorcluster)  [unwired: 6 in, 2 out]
        n148 = Concatenate Strings(w369, " " ("string"), w368) -> (→"Status":string)
      }
      frame Default {
        # "Call this case if a message is received that is not handled \nby any other case. Typically this is a programming error\nas a result of a typo or unhandled message/missing message handler."
        n149 = Format Into String(format string="DevError: Missing message handler for '%s\" message." ("message"), w374) -> (resulting string=w372:string)  [unwired: 2 in, 1 out]
        n150 = One Button Dialog(message=w372) -> ()  [unwired: 1 in, 1 out]
      }
      frame "Initialize" {
        w378 = u32 115200 ("baud rate (9600)")
        # "Initialize the state variables and user interface\nInitialize serial connections"
        n151 = call-poly "VISA Configure Serial Port"("VISA resource name"=w387, "baud rate (9600)"=w378, "error in (no error)"=w386) -> ("error out"=w385:errorcluster)  [unwired: 11 in, 1 out]
        n152 = call-poly "VISA Configure Serial Port"("VISA resource name"=w384, "baud rate (9600)"=w378, "error in (no error)"=w385) -> ("error out"=w382:errorcluster)  [unwired: 11 in, 1 out]
        n153 = call-poly "VISA Configure Serial Port"("VISA resource name"=w383, "baud rate (9600)"=w378, "error in (no error)"=w382) -> ("error out"=w377:errorcluster)  [unwired: 11 in, 1 out]
        n154 = call-poly "VISA Configure Serial Port"("VISA resource name"=w379, "baud rate (9600)"=w378, "error in (no error)"=w377) -> ("error out"=w376:errorcluster)  [unwired: 11 in, 1 out]
        n155 = call-poly "VISA Configure Serial Port"("VISA resource name"=w381, "error in (no error)"=w376) -> ("error out"=w380:errorcluster)  [unwired: 12 in, 1 out]
      }
      frame "sweep" {
        # "Perform a frequency sweep and calculate the resonance frequency"
        n156 = stacked-sequence {
          seq-local: [_ w413 _ _] -> [_ _ w439 _]
          tunnel: w398 -> [_ w407 _ _]
          tunnel: "End (Hz)" -> [_ w410 w430 _]
          tunnel: "Start (Hz)" -> [_ w409 w429 _]
          tunnel: w397 -> [w403 _ _ w448]
          tunnel: w394 -> [_ _ _ _]
          tunnel: w393 -> [_ w408 _ _]
          tunnel: w392 -> [_ _ _ w453]
          tunnel: [_ _ _ w450] -> w391
          tunnel: w390 -> [w404 _ _ w449]
          tunnel: w389 -> [w400 _ _ w444]
          frame #0 {
            w401 = FALSE
            # "Turn red, green, and IR lasers off for scan."
            n157 = call "laserOnOff.vi"("Emission (F = OFF)"=w401, "VISA Refnum in"=w404) -> ("error out"=w406:errorcluster)  [unwired: 7 in, 2 out]
            n158 = Wait (ms)(milliseconds to wait=u32 5000) -> ()  [unwired: 1 out]
            n159 = call "laserOnOff.vi"("error in (no error)"=w406, "Emission (F = OFF)"=w401, "VISA Refnum in"=w403) -> ("error out"=w402:errorcluster)  [unwired: 6 in, 2 out]
            n160 = call "laserOnOff.vi"("error in (no error)"=w402, "Emission (F = OFF)"=w401, "VISA Refnum in"=w400) -> ()  [unwired: 6 in, 3 out]
          }
          frame #1 {
            n161 = Subtract(x=w410, y=w409) -> (x-y=w411:i32)
            n162 = for {
              N: w411 -> [_]
              tunnel: [w419] -> w413 mode=indexing
              tunnel: w409 -> [w418]
              tunnel: w410 -> [w417]
              tunnel: w407 -> [_]
              i -> [w416]
              # "Get microphone data."
              # "Listen for N*2000\n seconds"
              n163 = local read "Mic FFT"() -> (w415:cluster{"f0":dbl, "df":dbl, "magnitude":dbl[]})
              n164 = Wait (ms)(milliseconds to wait=u32 2000) -> ()  [unwired: 1 out]
              n165 = Unbundle By Name(w415) -> ("magnitude"=w414:dbl[])
              n166 = call "fftGetMax.vi"("End Frequency (Hz)"=w417, "Start Frequency (Hz)"=w418, "Magnitudes"=w414) -> ("max value"=w419:dbl)  [unwired: 8 in]
              "Step No." <- w416
            }
            n167 = case shown="True" "sweep laser?" {
              tunnel: w409 -> [_ w426]
              tunnel: w410 -> [_ w425]
              tunnel: w408 -> [_ w424]
              tunnel: [w421 w423] -> _
              tunnel: w407 -> [w421 w422]
              frame False {
              }
              frame True {
                # "Scan laser freq.\nwith Teensy"
                n168 = call "teensySweepFreq.vi"("error in (no error)"=w422, "end f, Hz (1385)"=w425, "start f, Hz (1355)"=w426, "VISA Refnum in"=w424) -> ("error out"=w423:errorcluster)  [unwired: 7 in]
              }
            }
          }
          frame #2 {
            # "Calculate resonance frequency;\ndisplay and save scan."
            n169 = Wait (ms)(milliseconds to wait=u32 5000) -> ()  [unwired: 1 out]
            n170 = To Double Precision Float(number=w430) -> (double precision float=w427:dbl)
            n171 = To Double Precision Float(number=w429) -> (double precision float=w428:dbl)
            n172 = call "resCalc.vi"("Frequency Sweep"=w439, "Start F, Hz (1355)"=w429) -> ("F-res, Hz"=w434:dbl, "Frequency Scan"=w436:cluster{i32[], "Best Gaussian Fit":dbl[]}[])  [unwired: 8 in]
            "Frequency Scan" <- w436
            n173 = In Range and Coerce(upper limit=w427, x=w434, lower limit=w428) -> (In Range?=w433:bool)  [unwired: 1 out]
            n174 = And(x=w433, y="check freqs?") -> (x .and. y?=w431:bool)
            n175 = case shown="True" "Save sweeps?" {
              tunnel: "Frequency Sweep File Path" -> [_ w443]
              tunnel: w436 -> [_ w442]
              tunnel: w434 -> [_ w441]
              frame False {
              }
              frame True {
                n176 = call "saveFreqSweep.vi"("f-res, Hz"=w441, "Frequency Scan"=w442, "file path (dialog if empty)"=w443) -> ()  [unwired: 9 in]
              }
            }
            n177 = case shown="True" w431 {
              tunnel: w434 -> [_ w440]
              frame False {
              }
              frame True {
                n178 = property on="Calculated Resonance (Hz)" class="DigNum (strict)"("Val(Sgnl)"=w440) -> ()  [unwired: 2 in, 2 out]
                "Calculated Resonance (Hz)" <- w440
              }
            }
          }
          frame #3 {
            w445 = TRUE
            # "Turn red and green lasers back on."
            n179 = call "laserOnOff.vi"("Emission (F = OFF)"=w445, "VISA Refnum in"=w449) -> ("error out"=w454:errorcluster)  [unwired: 7 in, 2 out]
            n180 = call "laserOnOff.vi"("error in (no error)"=w454, "Emission (F = OFF)"=w445, "VISA Refnum in"=w448) -> ("error out"=w447:errorcluster)  [unwired: 6 in, 2 out]
            n181 = call "laserOnOff.vi"("error in (no error)"=w447, "Emission (F = OFF)"=w445, "VISA Refnum in"=w444) -> ("error out"=w446:errorcluster)  [unwired: 6 in, 2 out]
            n182 = call-poly "QMH Add Message to Queue.vi"("error in (no error)"=w446, "Parameter"="532 F (Hz)", "Message"="freqset", "queue in"=w453) -> ("error out"=w450:errorcluster)  [unwired: 6 in, 1 out]
          }
        }
      }
      frame "freqset" {
        # "Set the frequency of the Teensy's modulation\nsignal for single laser (if single frequency is changed)."
        # "Set the laser frequency.  Case for \"red\", \"blue\", or \"green\"."
        n183 = case shown="\"785 F (Hz)\"" w455 {
          tunnel: w457 -> [w464 w469 w474 w479]
          tunnel: [w463 w468 w473 w478] -> w456
          tunnel: w458 -> [w461 w466 w471 w477]
          frame "405 F (Hz) ", Default {
            w460 = u16 0 items=["blue", "green", "red", "ir"] ("laser")
            n184 = call "freqSet.vi"("error in (no error)"=w464, "laser"=w460, "Freq, Hz (1370)"="405 F (Hz)", "Teensy Port"=w461) -> ("error out"=w463:errorcluster)  [unwired: 6 in, 1 out]
          }
          frame "532 F (Hz)" {
            w465 = u16 1 items=["blue", "green", "red", "ir"] ("laser")
            n185 = call "freqSet.vi"("error in (no error)"=w469, "laser"=w465, "Freq, Hz (1370)"="532 F (Hz)", "Teensy Port"=w466) -> ("error out"=w468:errorcluster)  [unwired: 6 in, 1 out]
          }
          frame "660 F (Hz)" {
            w470 = u16 2 items=["blue", "green", "red", "ir"] ("laser")
            n186 = call "freqSet.vi"("error in (no error)"=w474, "laser"=w470, "Freq, Hz (1370)"="660 F (Hz)", "Teensy Port"=w471) -> ("error out"=w473:errorcluster)  [unwired: 6 in, 1 out]
          }
          frame "785 F (Hz)" {
            w475 = u16 3 items=["blue", "green", "red", "ir"] ("laser")
            n187 = call "freqSet.vi"("error in (no error)"=w479, "laser"=w475, "Freq, Hz (1370)"="785 F (Hz)", "Teensy Port"=w477) -> ("error out"=w478:errorcluster)  [unwired: 6 in, 1 out]
          }
        }
      }
      frame "setfreqs" {
        # "Set the frequency of the Teensy's modulation\nsignal for all lasers at once."
        # "Set laser frequencies to resonance frequency calculated in sweep."
        n188 = Scan From String(input string=w480, error in=w482) -> (error out=w481:errorcluster, output 1=w483:dbl)  [unwired: 3 in, 2 out]
        n189 = for {
          N: 4 -> [_]
          tunnel: [w493] -> w484
          tunnel: w481 -> [w492]
          tunnel: w485 -> [w489]
          tunnel: w483 -> [w491]
          i -> [w490]
          n190 = flat-sequence {
            tunnel: w489 -> [w494]
            tunnel: [w494] -> w488
            frame #0 {
              n191 = Wait (ms)(milliseconds to wait=u32 1000) -> ()  [unwired: 1 out]
            }
          }
          n192 = case shown="0, Default" w490 {
            tunnel: [w503 w511 w519 w527] -> w493
            tunnel: w492 -> [w501 w509 w517 w524]
            tunnel: w488 -> [w500 w508 w516 w523]
            tunnel: w491 -> [w497 w505 w513 w520]
            frame 0, Default {
              w496 = u16 2 items=["blue", "green", "red", "ir"] ("laser")
              n193 = Add(x=w497, y=1.0) -> (x+y=w499:dbl)
              n194 = To Long Integer(number=w499) -> (32bit integer=w498:i32)
              n195 = call "freqSet.vi"("error in (no error)"=w501, "laser"=w496, "Freq, Hz (1370)"=w498, "Teensy Port"=w500) -> ("error out"=w503:errorcluster)  [unwired: 6 in, 1 out]
              n196 = local write "660 F (Hz)"(w498) -> ()
            }
            frame 1 {
              w504 = u16 3 items=["blue", "green", "red", "ir"] ("laser")
              n197 = Subtract(x=w505, y=1.0) -> (x-y=w507:dbl)
              n198 = To Long Integer(number=w507) -> (32bit integer=w506:i32)
              n199 = call "freqSet.vi"("error in (no error)"=w509, "laser"=w504, "Freq, Hz (1370)"=w506, "Teensy Port"=w508) -> ("error out"=w511:errorcluster)  [unwired: 6 in, 1 out]
              n200 = local write "785 F (Hz)"(w506) -> ()
            }
            frame 2 {
              w512 = u16 0 items=["blue", "green", "red", "ir"] ("laser")
              n201 = Subtract(x=w513, y=2.0) -> (x-y=w515:dbl)
              n202 = To Long Integer(number=w515) -> (32bit integer=w514:i32)
              n203 = call "freqSet.vi"("error in (no error)"=w517, "laser"=w512, "Freq, Hz (1370)"=w514, "Teensy Port"=w516) -> ("error out"=w519:errorcluster)  [unwired: 6 in, 1 out]
              n204 = local write "405 F (Hz)"(w514) -> ()
            }
            frame 3 {
              w526 = u16 1 items=["blue", "green", "red", "ir"] ("laser")
              n205 = Add(x=w520, y=2.0) -> (x+y=w522:dbl)
              n206 = To Long Integer(number=w522) -> (32bit integer=w521:i32)
              n207 = call "freqSet.vi"("error in (no error)"=w524, "laser"=w526, "Freq, Hz (1370)"=w521, "Teensy Port"=w523) -> ("error out"=w527:errorcluster)  [unwired: 6 in, 1 out]
              n208 = local write "532 F (Hz)"(w521) -> ()
            }
          }
        }
      }
      frame "405 emit" {
        # "Turn laser on or off"
        n209 = call "laserOnOff.vi"("error in (no error)"=w532, "Emission (F = OFF)"="405 Emission", "Power, mW (100)"="405 Power (mW)", "VISA Refnum in"=w531) -> ("error out"=w528:errorcluster)  [unwired: 5 in, 2 out]
      }
      frame "532 emit" {
        # "Turn laser on or off"
        n210 = call "laserOnOff.vi"("error in (no error)"=w538, "Emission (F = OFF)"="532 Emission", "Power, mW (100)"="532 Power (mW)", "VISA Refnum in"=w535) -> ("error out"=w534:errorcluster)  [unwired: 5 in, 2 out]
      }
      frame "660 emit" {
        # "Turn laser on or off"
        n211 = call "laserOnOff.vi"("error in (no error)"=w544, "Emission (F = OFF)"="660 Emission", "Power, mW (100)"="660 Power (mW)", "VISA Refnum in"=w541) -> ("error out"=w540:errorcluster)  [unwired: 5 in, 2 out]
      }
      frame "785 emit" {
        # "Turn laser on or off"
        n212 = call "laserOnOff.vi"("error in (no error)"=w551, "Emission (F = OFF)"="785 Emission", "Power, mW (100)"="785 Power (mW)", "VISA Refnum in"=w546) -> ("error out"=w549:errorcluster)  [unwired: 5 in, 2 out]
      }
      frame "emit" {
        # "Turn on all lasers."
        n213 = local write "405 Emission"("All Emit") -> ()
        n214 = local write "532 Emission"("All Emit") -> ()
        n215 = local write "660 Emission"("All Emit") -> ()
        n216 = local write "785 Emission"("All Emit") -> ()
      }
      frame "405 Power" {
        # "Set laser power"
        n217 = Scan From String(input string=w558, error in=w556) -> (error out=w555:errorcluster, output 1=w557:dbl)  [unwired: 3 in, 2 out]
        n218 = call "laserSetPower.vi"("error in (no error)"=w555, "Laser Power (mW)"=w557, "VISA Refnum in"=w561) -> ("error out"=w559:errorcluster)  [unwired: 7 in, 1 out]
      }
      frame "532 Power" {
        n219 = Scan From String(input string=w562, error in=w565) -> (error out=w564:errorcluster, output 1=w563:dbl)  [unwired: 3 in, 2 out]
        n220 = call "laserSetPower.vi"("error in (no error)"=w564, "Laser Power (mW)"=w563, "VISA Refnum in"=w567) -> ("error out"=w566:errorcluster)  [unwired: 7 in, 1 out]
      }
      frame "660 Power" {
        n221 = Scan From String(input string=w569, error in=w572) -> (error out=w571:errorcluster, output 1=w570:dbl)  [unwired: 3 in, 2 out]
        n222 = call "laserSetPower.vi"("error in (no error)"=w571, "Laser Power (mW)"=w570, "VISA Refnum in"=w574) -> ("error out"=w573:errorcluster)  [unwired: 7 in, 1 out]
      }
      frame "785 Power" {
        n223 = Scan From String(input string=w576, error in=w579) -> (error out=w578:errorcluster, output 1=w577:dbl)  [unwired: 3 in, 2 out]
        n224 = call "laserSetPower.vi"("error in (no error)"=w578, "Laser Power (mW)"=w577, "VISA Refnum in"=w581) -> ("error out"=w580:errorcluster)  [unwired: 7 in, 1 out]
      }
      frame "align" {
        # "Set power of all lasers to 5 mW for alignment"
        n225 = case shown="False" "Alignment Mode" {
          tunnel: w588 -> [w600 w613]
          tunnel: w587 -> [w599 w612]
          tunnel: w586 -> [w598 w611]
          tunnel: w585 -> [w597 w610]
          tunnel: [w591 w602] -> w584
          tunnel: w583 -> [w592 w603]
          frame True {
            w593 = 5.0 ("Laser Power (mW)")
            n226 = call "laserSetPower.vi"("error in (no error)"=w600, "Laser Power (mW)"=w593, "VISA Refnum in"=w599) -> ("error out"=w596:errorcluster)  [unwired: 7 in, 1 out]
            n227 = call "laserSetPower.vi"("error in (no error)"=w596, "Laser Power (mW)"=w593, "VISA Refnum in"=w598) -> ("error out"=w595:errorcluster)  [unwired: 7 in, 1 out]
            n228 = call "laserSetPower.vi"("error in (no error)"=w595, "Laser Power (mW)"=w593, "VISA Refnum in"=w597) -> ("error out"=w594:errorcluster)  [unwired: 7 in, 1 out]
            n229 = call "laserSetPower.vi"("error in (no error)"=w594, "Laser Power (mW)"=w593, "VISA Refnum in"=w592) -> ("error out"=w591:errorcluster)  [unwired: 7 in, 1 out]
          }
          frame False, Default {
            n230 = local read "405 Power (mW)"() -> (w607:dbl)
            n231 = local read "532 Power (mW)"() -> (w606:dbl)
            n232 = local read "660 Power (mW)"() -> (w605:dbl)
            n233 = local read "785 Power (mW)"() -> (w604:dbl)
            n234 = call "laserSetPower.vi"("error in (no error)"=w613, "Laser Power (mW)"=w607, "VISA Refnum in"=w612) -> ("error out"=w609:errorcluster)  [unwired: 7 in, 1 out]
            n235 = call "laserSetPower.vi"("error in (no error)"=w609, "Laser Power (mW)"=w606, "VISA Refnum in"=w611) -> ("error out"=w608:errorcluster)  [unwired: 7 in, 1 out]
            n236 = call "laserSetPower.vi"("error in (no error)"=w608, "Laser Power (mW)"=w605, "VISA Refnum in"=w610) -> ("error out"=w601:errorcluster)  [unwired: 7 in, 1 out]
            n237 = call "laserSetPower.vi"("error in (no error)"=w601, "Laser Power (mW)"=w604, "VISA Refnum in"=w603) -> ("error out"=w602:errorcluster)  [unwired: 7 in, 1 out]
          }
        }
      }
      frame "background" {
        n238 = local read "mic ts"() -> (w614:T3)
        n239 = local write "Bkg Values (mV)"(w614) -> ()
      }
      frame "filter" {
        n240 = local read "Filtering"() -> (w621:bool)
        n241 = case shown="True" w621 {
          tunnel: w620 -> [w625 w634]
          tunnel: w619 -> [w624 w632]
          tunnel: [w623 w633] -> w618
          frame False {
            n242 = Multiply(x="Filter Length (min)", y=60.0) -> (x*y=w628:dbl)
            n243 = local write "Time Target (s)"(w628) -> ()
            n244 = VISA Write(VISA resource name=w625, write buffer="v.1", error in (no error)=w624) -> (error out=w623:errorcluster)  [unwired: 2 out]
            "Filtering" <- TRUE
          }
          frame True {
            n245 = flat-sequence {
              tunnel: w632 -> [w641]
              tunnel: [w641] -> w631
              frame #0 {
                n246 = local read "mic ts"() -> (w640:T3)
                n247 = local write "Bkg Values (mV)"(w640) -> ()
              }
            }
            n248 = local write "Filtering"(FALSE) -> ()
            n249 = VISA Write(VISA resource name=w634, write buffer="v.0", error in (no error)=w631) -> (error out=w633:errorcluster)  [unwired: 2 out]
            n250 = Multiply(x="Sample Length (min)", y=60.0) -> (x*y=w636:dbl)
            n251 = local write "Time Target (s)"(w636) -> ()
          }
        }
        n252 = Wait (ms)(milliseconds to wait=u32 500) -> ()  [unwired: 1 out]
      }
      frame "filterswitch" {
        n253 = case shown="\"TRUE\"" w642 {
          tunnel: w645 -> [w649 w654]
          tunnel: w644 -> [w648 w653]
          tunnel: [w647 w652] -> w643
          frame "FALSE", Default {
            n254 = VISA Write(VISA resource name=w649, write buffer="v.0", error in (no error)=w648) -> (error out=w647:errorcluster)  [unwired: 2 out]
          }
          frame "TRUE" {
            n255 = VISA Write(VISA resource name=w654, write buffer="v.1", error in (no error)=w653) -> (error out=w652:errorcluster)  [unwired: 2 out]
          }
        }
      }
      frame "calibrate" {
        n256 = control-ref of="aligned data"() -> (w683:refnum<vi>)
        n257 = call "go3Import.vi"("go3 data"="GO3 Filepath") -> ("flows, sccm"=w685:dbl[][], "[o3], ppb"=w684:dbl[][])  [unwired: 9 in]
        n258 = call "micImport.vi"("mic data"="Microphone Filepath") -> ("mic data"=w675:cluster{dbl[][], dbl[][]})  [unwired: 8 in, 2 out]
        n259 = call "pdImport.vi"("pd data"="Photodiode Filepath") -> ("pd data"=w676:cluster{dbl[][], dbl[][]})  [unwired: 8 in, 2 out]
        n260 = property class="XYGraph (strict)"(reference=w683) -> ("CrsrList"=w682:T12)  [unwired: 1 in, 2 out]
        n261 = call "calNormalize.vi"("532 pd Cal"="532 PD Cal", "660 pd Cal"="660 PD Cal", "pd data"=w676, "mic data"=w675) -> ("660 Normalized"=w679:dbl[], "532 Normalized"=w680:dbl[])  [unwired: 6 in]
        n262 = call "calConvertToND.vi"("O3 Flow, sccm (80)"="O3 Flow, sccm (80)", "flows, sccm"=w685, "[o3], ppb"=w684) -> ("Array"=w670:dbl[])  [unwired: 8 in]
        n263 = call "calDecimateTS.vi"("660 Data"=w679, "532 Data"=w680) -> ("Decimated 660"=w672:dbl[], "Decimated 532"=w671:dbl[])  [unwired: 8 in]
        n264 = call "calSubtractBkg.vi"("bkg end"="Bkg End Index", "bkg start"="Bkg Start Index", "660"=w672, "532"=w671) -> ("660 Substracted"=w663:dbl[], "532 Subtracted"=w664:dbl[])  [unwired: 6 in]
        n265 = call "calSubset.vi"("offset"="GO3 Offset", "CrsrList"=w682, "Decimated 660"=w663, "Decimated 532"=w664, "GO3 Data"=w670) -> ("660 Subset"=w661:dbl[], "532 Subset"=w662:dbl[], "Go3 Subset"=w669:dbl[])  [unwired: 4 in]
        n266 = call "calAlign.vi"("offset"="GO3 Offset", "Decimated 660"=w663, "Decimated 532"=w664, "GO3 Data"=w670) -> ("Aligned Data"=→"aligned data":cluster{"Array":i32[], "Decimated 660":dbl[]}[])  [unwired: 7 in]
        n267 = call "calLinFit.vi"("660 Subset"=w661, "532 Subset"=w662, "Go3 Subset"=w669) -> ("cal coef"=→"PAS Cal Coefficient":dbl, "660 Slope"=w658:dbl, "532 slope"=w659:dbl, "Calibration"=w657:cluster{dbl[], "Best Linear Fit":dbl[]}[])  [unwired: 5 in]
        "Calibration" <- w657
        "532 Slope" <- w659
        "660 Slope" <- w658
        n268 = call "calSave.vi"("O3 flow"="O3 Flow, sccm (80)", "save cal?"="Save Cal?", "m_660"=w658, "m_532"=w659, "Calibration"=w657, "file path (dialog if empty)"="Calibration Filepath") -> ()  [unwired: 6 in]
      }
      frame "Error" {
        (unwired) errorcluster {"status"=FALSE, "code"=0, "source"=""} ("error out")
        # "Proceed to Exit - remove if this is\nnot appropriate for the General Error case"
        # "General Error Case - this case is called if an error is passed using the error cluster below. Typically most new errors should be handed in each individual case and not passed in the rror cluster. If necessary a custom error handler case should be added and called from other cases."
        n269 = call <vilib>:"Simple Error Handler.vi"("error in (no error)"=w693) -> ("error out"=w689:errorcluster)  [unwired: 4 in, 4 out]
        n270 = call-poly "QMH Add Message to Queue.vi"("error in (no error)"=w689, "Message"="Exit", "queue in"=w692) -> ("error out"=w690:errorcluster)  [unwired: 7 in, 1 out]
      }
      frame "Exit" {
        # "Perform cleanup tasks: Close serial connections and clear front panel."
        n271 = call "QMH Destroy Queue.vi"("error in (no error)"=w708, "queue in"=w707) -> ("error out"=w700:errorcluster)  [unwired: 7 in, 2 out]
        n272 = for {
          N: 4 -> [_]
          tunnel: w703 -> [w716]
          tunnel: w702 -> [w714]
          tunnel: w701 -> [w713]
          tunnel: w700 -> [w712]
          tunnel: FALSE -> [w711]
          tunnel: [w710] -> w696
          tunnel: w695 -> [w709]
          i -> [w715]
          # "Close laser serial connections."
          n273 = case shown="3" w715 {
            tunnel: [w723 w728 w733 w738] -> w718
            tunnel: [w722 w727 w732 w737] -> w717
            tunnel: w716 -> [w721 _ _ _]
            tunnel: w714 -> [_ w726 _ _]
            tunnel: w713 -> [_ _ _ w735]
            tunnel: w712 -> [w720 w725 w731 w736]
            tunnel: w711 -> [w719 w724 w730 w734]
            tunnel: w709 -> [_ _ w729 _]
            frame 0, Default {
              n274 = call "laserOnOff.vi"("error in (no error)"=w720, "Emission (F = OFF)"=w719, "VISA Refnum in"=w721) -> ("error out"=w723:errorcluster, "VISA Refnum out"=w722:refnum<visa-resource-name>)  [unwired: 6 in, 1 out]
              n275 = local write "405 Emission"(w719) -> ()
            }
            frame 1 {
              n276 = call "laserOnOff.vi"("error in (no error)"=w725, "Emission (F = OFF)"=w724, "VISA Refnum in"=w726) -> ("error out"=w728:errorcluster, "VISA Refnum out"=w727:refnum<visa-resource-name>)  [unwired: 6 in, 1 out]
              n277 = local write "532 Emission"(w724) -> ()
            }
            frame 2 {
              n278 = call "laserOnOff.vi"("error in (no error)"=w731, "Emission (F = OFF)"=w730, "VISA Refnum in"=w729) -> ("error out"=w733:errorcluster, "VISA Refnum out"=w732:refnum<visa-resource-name>)  [unwired: 6 in, 1 out]
              n279 = local write "785 Emission"(w730) -> ()
            }
            frame 3 {
              n280 = call "laserOnOff.vi"("error in (no error)"=w736, "Emission (F = OFF)"=w734, "VISA Refnum in"=w735) -> ("error out"=w738:errorcluster, "VISA Refnum out"=w737:refnum<visa-resource-name>)  [unwired: 6 in, 1 out]
              n281 = local write "660 Emission"(w734) -> ()
              n282 = local write "All Emit"(w734) -> ()
            }
          }
          n283 = VISA Close(VISA resource name=w717, error in (no error)=w718) -> (error out=w710:errorcluster)
        }
        n284 = local write "Status"("" ("Status")) -> ()
        n285 = VISA Close(VISA resource name=w704, error in (no error)=w696) -> (error out=w697:errorcluster)
      }
    }
    n286 = case shown="True" "Auto Filter" {
      tunnel: [w347 w349] -> w331
      tunnel: w330 -> [w347 w348]
      frame False {
      }
      frame True {
        # "This is the timer for the filtering routine."
        n287 = call "Elapsed Time"("Time Target (s)"="Time Target (s)", "Auto Reset"=TRUE, "error in (no error)"=w348) -> ("Elapsed Time (s)"=w352:dbl, "Time has Elapsed"=w354:bool, "error out"=w353:errorcluster)  [unwired: 9 in, 5 out]
        "Time has Elapsed" <- w354
        n288 = Divide(x=w352, y=60.0) -> (x/y=→"Elapsed Time (min)":dbl)
        n289 = property on="Time has Elapsed" class="Bool (strict)"(error in=w353, "Val(Sgnl)"=w354) -> (error out=w349:errorcluster)  [unwired: 1 in, 1 out]
      }
    }
  }
  n290 = Merge Errors(w63, w54) -> (w62:errorcluster)
  n291 = call <vilib>:"Simple Error Handler.vi"("error in (no error)"=w62) -> ("error out"=w61:errorcluster)  [unwired: 4 in, 4 out]
  n292 = Release Queue(queue=w11, error in (no error)=w10) -> ()  [unwired: 1 in, 3 out]
  n293 = Release Queue(queue=w8, error in (no error)=w7) -> ()  [unwired: 1 in, 3 out]
  n294 = flat-sequence {
    tunnel: w61 -> [w739]
    tunnel: [w739] -> w60
    frame #0 {
      n295 = local write "Exit"(FALSE) -> ()
    }
  }
  "error out" <- w60
